vi "Interfaz grafica - corriente.vi"() -> ()   [LabVIEW 2024]
uses:
  160620 Optotune Lens Driver 4 Labview package/Hello Optotune Lens (30.06.2015)/Calibration.ctl
  <vilib>/DAQmx/read.llb/DAQmx Read (Analog 1D Wfm NChan NSamp).vi
  <vilib>/Analysis/2dsp.llb/Decimate (single shot, DBL).vi
  <vilib>/Utility/file.llb/Read Delimited Spreadsheet (string).vi
  <vilib>/Analysis/2dsp.llb/Decimate (continuous, DBL).vi
  <vilib>/Instr/_visa.llb/VISA Configure Serial Port (Instr).vi
  <vilib>/Utility/file.llb/Write Delimited Spreadsheet (string).vi
  <vilib>/DAQmx/create/channels.llb/DAQmx Create Channel (AI-Voltage-Basic).vi
  <vilib>/DAQmx/configure/timing.llb/DAQmx Timing (Sample Clock).vi
  <vilib>/DAQmx/miscellaneous.llb/DAQmx Fill In Error Info.vi
  <vilib>/Waveform/WDTOps.llb/WDT Index Channel DBL.vi
  <vilib>/Waveform/WDTOps.llb/WDT Get Waveform Time Array DBL.vi
  <vilib>/Analysis/NI_AALPro.lvlib
panel:
  out "Array 4":string[](array[string])
  out "Array 3":string[](array[string])
  out "Array 2":string[](array[string])
  out "Array":string[](array[string])
  out "Nombre 2":string
  in  "Restablecer Iniciales":bool
  in  "Incremento":dbl=0.1 format="%#_13g"
  out "Potencia derecho":dbl
  out "error out 4":errorcluster
  out "error out 3":errorcluster
  out "error out 2":errorcluster
  in  "Tab Control 3":enum32{"WL", "Video"}(tab)
  out "Waveform length":dbl[][](graph)
  in  "Minimo escala Y":dbl format="%#_13g"
  in  "Maximo escala Y":dbl format="%#_13g"
  in  "Escala autom. Y":u8=1
  in  "Escala autom. X":u8=1
  in  "Maximo escala X":dbl
  in  "Minimo escala X":dbl
  out "Image Out":T1(plugin-control)
  in  "Frame Rate":u32=30
  in  "Modo de video":u16(ring)=21 items=["160x90 I420 30 fps", "160x90 MJPG 30 fps", "160x90 RGB24 30 fps", "160x120 I420 30 fps", "160x120 MJPG 30 fps", "160x120 RGB24 30 fps", "176x144 I420 30 fps", "176x144 MJPG 30 fps", "176x144 RGB24 30 fps", "320x180 I420 30 fps", "320x180 MJPG 30 fps", "320x180 RGB24 30 fps", "320x240  I420 30 fps", "320x240 MJPG 30 fps", "320x240 RGB24 30 fps", "352x288 I420 30 fps", "352x288 MJPG 30 fps", "352x288 RGB24 30 fps", "432x240 I420 30 fps", "432x240 MJPG 30 fps", "432x240 RGB24 30 fps", "640x360 I420 30 fps", "640x360 MJPG 30 fps", "640x360 RGB24 30 fps", "640x480 I420 30 fps", "640x480 MJPG 30 fps", "640x480 RGB24 30 fps", "800x448 I420 30 fps", "800x448 MJPG 30 fps", "800x448 RGB24 30 fps", "800x600 I420 30 fps", "800x600 MJPG 30 fps", "800x600 RGB24 30 fps", "864x480 I420 30 fps", "864x480 MJPG 30 fps", "864x480 RGB24 30 fps", "960x720 I420 30 fps", "960x720 MJPG 30 fps", "960x720 RGB24 30 fps", "1024x576 I420 30 fps", "1024x576 MJPG 30 fps", "1024x576 RGB24 30 fps", "1280x720 I420 30 fps", "1280x720 MJPG 30 fps", "1280x720 RGB24 30 fps", "1600x896 I420 30 fps", "1600x896 MJPG 30 fps", "1600x896 RGB24 30 fps", "1920x1080 I420 5 fps", "1920x1080 MJPG 30 fps", "1920x1080 RGB24 5 fps", "2304x1296 I420 2 fps", "2304x1296 RGB24 2 fps", "2304x1536 I420 2 fps", "2304x1536 RGB24 2 fps"]
  in  "Carpeta archivo":string="C:\\Users\\TGM1603\\Documents\\LabVIEW Data\\Experimentos electrodos\\VideosExperimentos"
  in  "Calidad":u32=1000
  out "VISA resource name out":string
  in  "Tab Control 2":T2(tab)
  in  "factor decimacion":i32=20
  in  "Ganancia":u16(ring) items=["0.2"=51455, "1"=33023, "10"=49407, "20"=41215, "30"=57599, "40"=37119, "60"=53503, "80"=45311, "120"=61695, "157"=35071, ""=0]
  in  "Potencia inicial lente derecho":dbl(slide) scale=-3.0..3.0
  in  "Potencia inicial lente izquierdo":dbl(slide) scale=-3.0..3.0
  in  "VISA resource name":string="COM11"
  in  "VISA resource name 2":string="COM10"
  out "DPT INICIALES D":dbl
  out "DPT INICIALES I":dbl
  out "Potencia izquierdo":dbl
  in  "error in (no error) 5":errorcluster
  in  "error in (no error) 4":errorcluster
  in  "error in (no error) 3":errorcluster
  in  "error in (no error) 2":errorcluster
  in  "Calibration 4":T3={"Max Current A"=293.0, "Max Current B"=293.0, "UCL A"=300.0, "UCL B"=300.0, "LCL A"=0.0, "LCL B"=0.0} {"Max Current A" format="%#_g mA"; "Max Current B" format="%#_g mA"; "UCL A" format="%#_g mA"; "LCL A" format="%#_g mA"; "UCL B" format="%#_g mA"; "LCL B" format="%#_g mA"}
  out "ID 2":u16
  out "VISA resource name out 2":string
  out "Calibration 3":T3 {"Max Current A" format="%#_g mA"; "Max Current B" format="%#_g mA"; "UCL A" format="%#_g mA"; "LCL A" format="%#_g mA"; "UCL B" format="%#_g mA"; "LCL B" format="%#_g mA"}
  out "OK 2":bool
  out "Data 2":string
  out "Command to Port 2":string
  in  "Cola tipo 2":dbl[](array[numeric])
  out "Distancia":u32
  in  "Tamaño ventana WL":i32=60
  in  "Limite inferior WL":dbl=25.0 format="%#_13g"
  in  "Limite superior WL":dbl=50.0
  out "number":u32
  in  "Calibration":T3={"Max Current A"=293.0, "Max Current B"=293.0, "UCL A"=300.0, "UCL B"=300.0, "LCL A"=0.0, "LCL B"=0.0} {"Max Current A" format="%#_g mA"; "Max Current B" format="%#_g mA"; "UCL A" format="%#_g mA"; "LCL A" format="%#_g mA"; "UCL B" format="%#_g mA"; "LCL B" format="%#_g mA"}
  out "ID":u16
  out "Calibration 2":T3 {"Max Current A" format="%#_g mA"; "Max Current B" format="%#_g mA"; "UCL A" format="%#_g mA"; "LCL A" format="%#_g mA"; "UCL B" format="%#_g mA"; "LCL B" format="%#_g mA"}
  out "OK":bool
  out "Data":string
  out "Command to Port":string
  in  "DPT dif.":dbl
  out "error out":errorcluster
  in  "error in (no error)":errorcluster
  in  "WL":dbl
  in  "Cola tipo":dbl[](array[numeric])
  out "T button?":bool
  in  "Elegir menu Exp":bool
  in  "Elegir menu":bool
  out "path":path
  in  "Iniciar experimento":bool
  in  "Parar adquisicion":bool
  out "Enfermedad visual":string
  out "Edad":string
  out "Nombre":string
  out "Cedula":string
  in  "Carpeta":path=path "C:/Users/TGM1603/Documents/LabVIEW Data/Experimentos electrodos"
  in  "?":bool
  in  "Menu Principal":u16(ring) items=["Visualizacion general ", "Llevar a cabo un experimento", "Ajustar potencia inicial lentes"]
  in  "Menu experimentos":u16(ring) items=["Experimento 1", "Experimento 2", "Experimento 3", "Experimento 4"]
  in  "Tab Control":enum32{"Señal EMG", "Potencia y distancia"}(tab)
  out "Senal EMG":waveform(dbl)[](graph)
  in  "Escala Y min":dbl
  in  "Escala Y max":dbl
  in  "Auto scale Y":u8=1
  in  "Escala X max":dbl
  in  "Escala X min":dbl
  out "Potencia optica y distancia":dbl[][](graph)
  in  "Auto scale X":u8=1
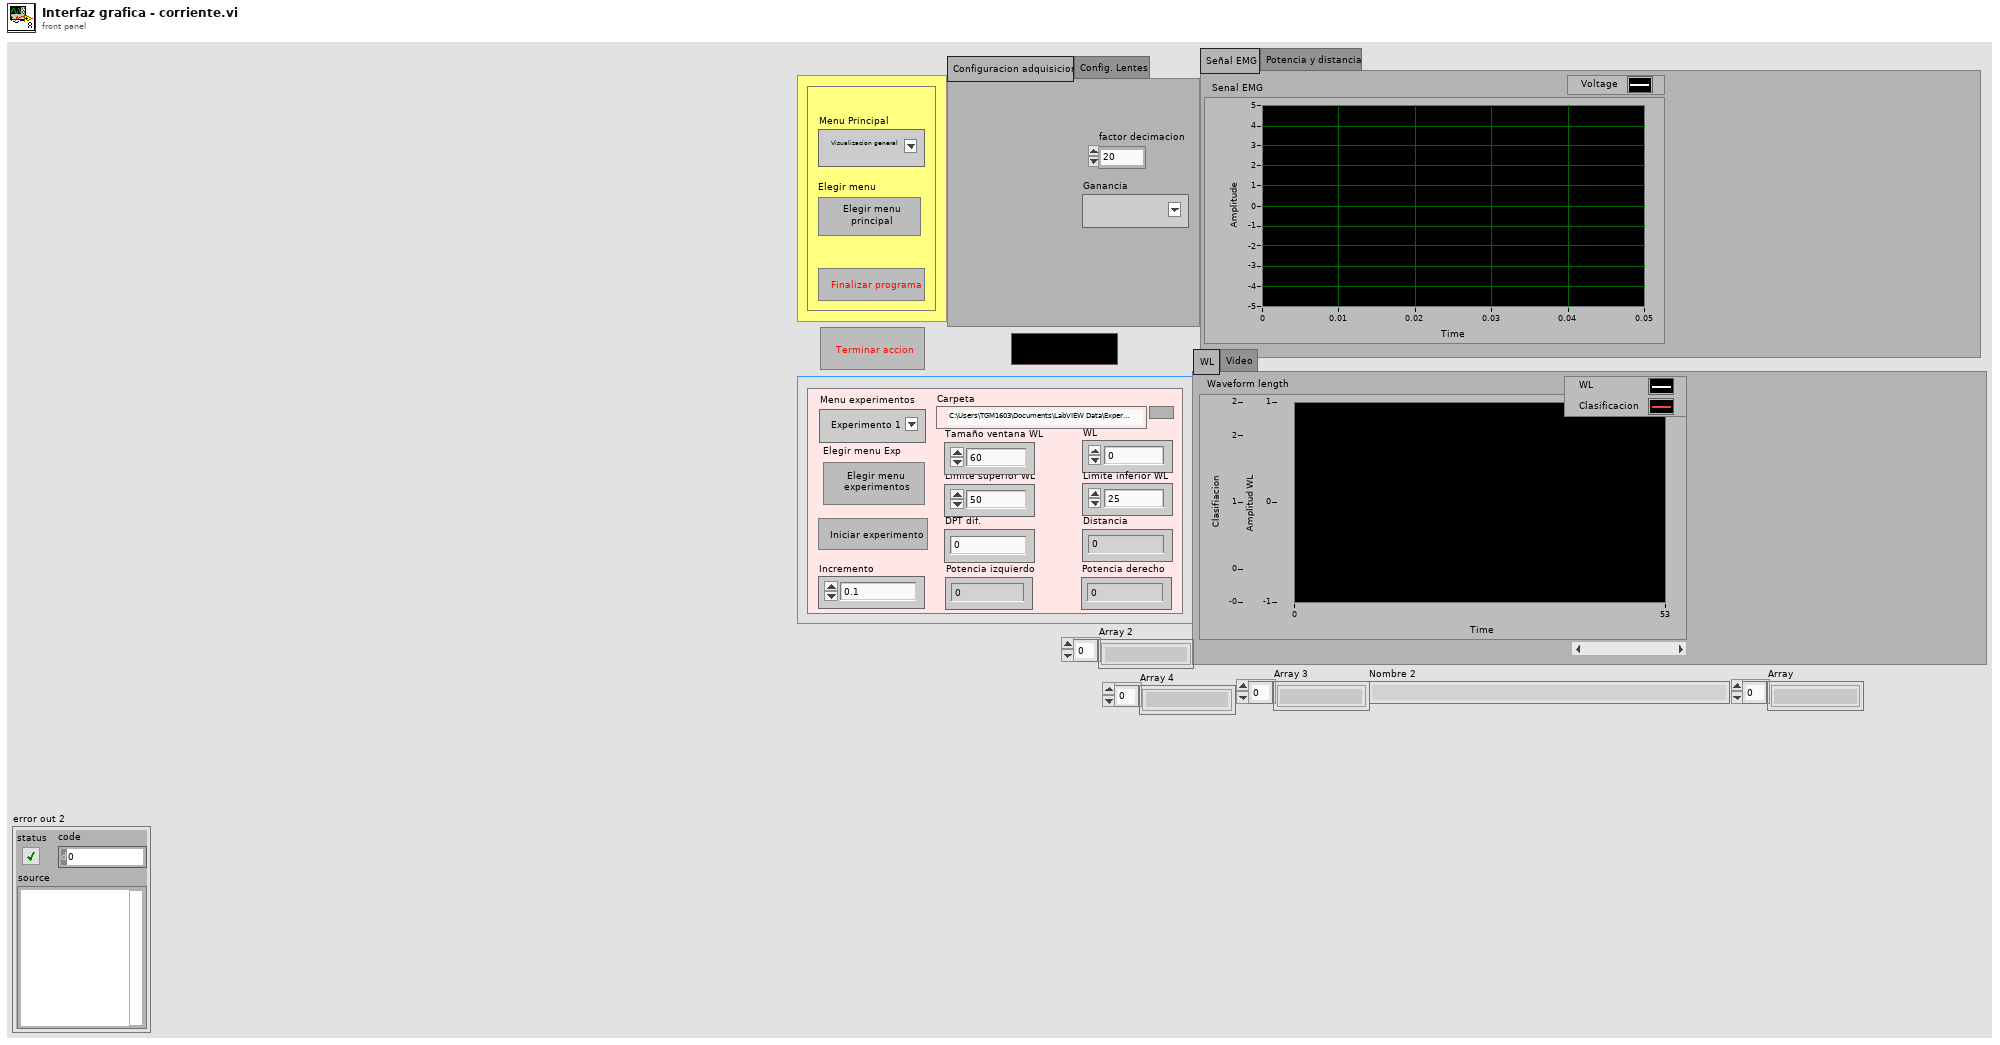
[diagram p1: front panel]
types:
  T1 = typedef "IMAQ Image.ctl" = refnum<image>
  T2 = enum32{"Configuracion adquisicion", "Config. Lentes"}
  T3 = typedef "Calibration.ctl" = cluster{"Max Current A":dbl, "Max Current B":dbl, "UCL A":dbl, "UCL B":dbl, "LCL A":dbl, "LCL B":dbl}
  T4 = enum16{"Left Button", "Center Button", "Right Button", "Window Close"}
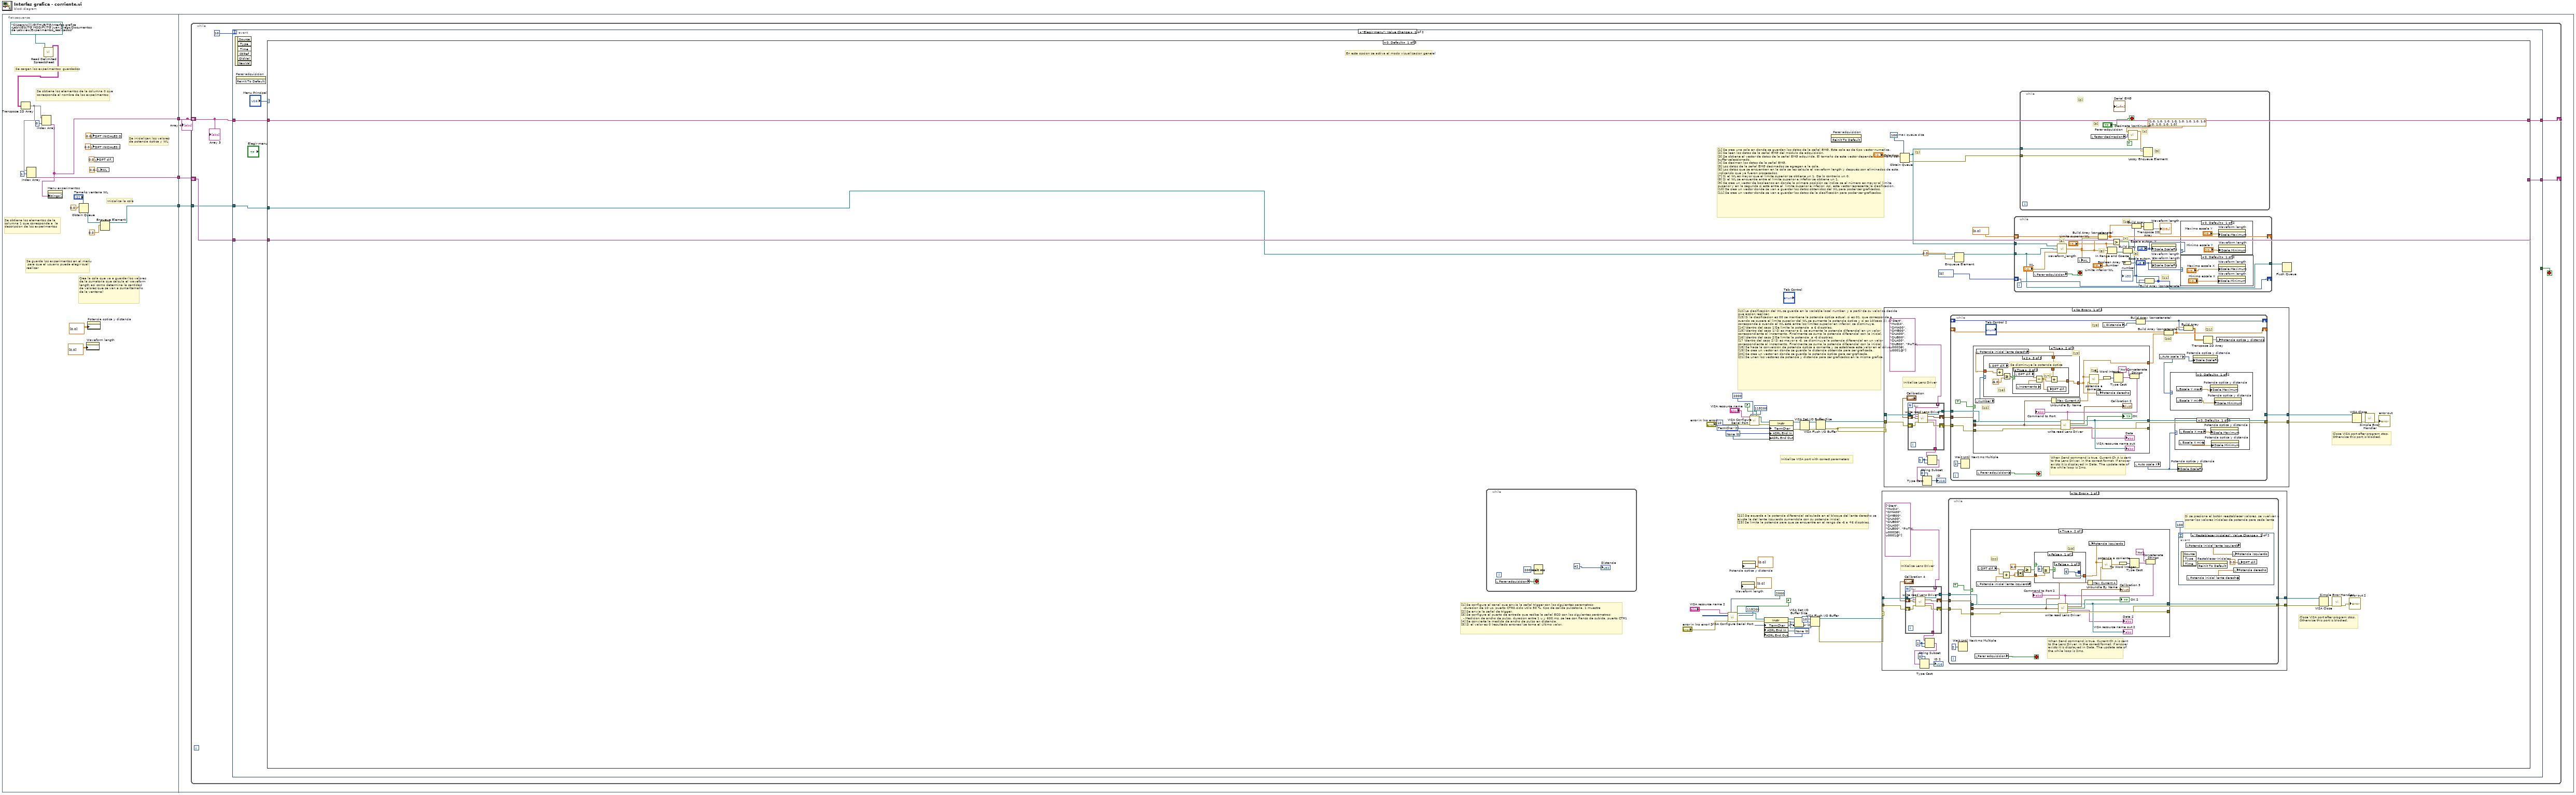
[diagram p0: block diagram]
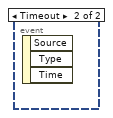
[diagram p2: hidden frame]
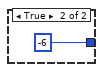
[diagram p4: hidden frame]
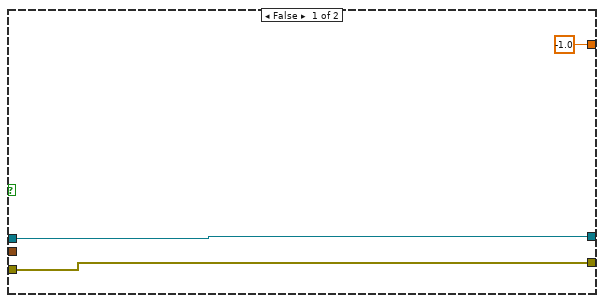
[diagram p9: hidden frame]
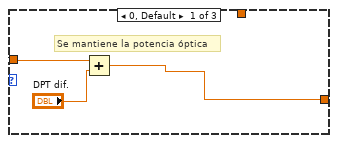
[diagram p10: hidden frame]
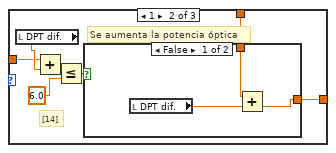
[diagram p11: hidden frame]
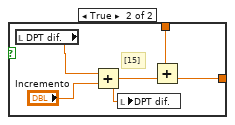
[diagram p12: hidden frame]
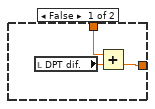
[diagram p13: hidden frame]
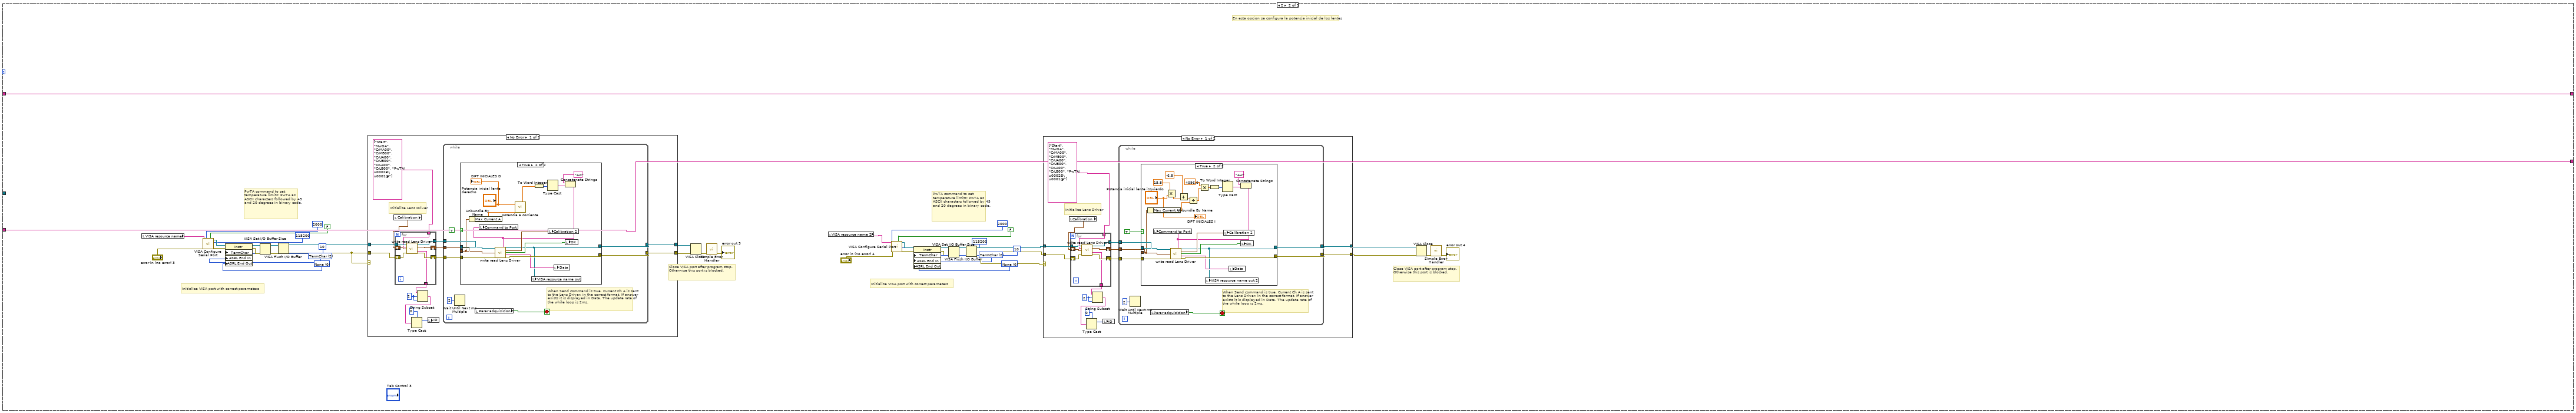
[diagram p17: hidden frame]
diagram:
  n1 = flat-sequence {
    tunnel: [w18] -> w3
    tunnel: [w15] -> w2
    tunnel: [w10] -> w1
    tunnel: w3 -> [w22]
    tunnel: w2 -> [w24]
    tunnel: w1 -> [w23]
    frame #0 {
      # "Se inicializan los valores\nde potencia óptica y WL"
      # "Inicializa la cola"
      # "Crea la cola que va a guardar los valores de la sumatoria que calcula el waveform length así como determina la cantidad de valores que se van a sumar(tamaño de la ventana)"
      # "Se obtiene los elementos de la columna 1 que corresponde a  la descripcion de los experimentos"
      # "Se obtiene los elementos de la columna 0 que corresponde al nombre de los experimentos"
      # "Se guarda los experimentos en el menu\n para que el usuario pueda elegir cual \nrealizar"
      # "Se cargan los experimentos  guardados"
      n2 = call-poly <vilib>:"Read Delimited Spreadsheet.vi"("file path (dialog if empty)"=path "C:/Users/willi/GITHUB/TG/Interfaz grafica -LabVIEW/TG MODIFY/TG Juan Diego/Documentos de Labview/Experimentos_realizados") -> ("all rows"=w19:string[][])  [unwired: 9 in, 5 out]
      n3 = Transpose 2D Array(2D array=w19) -> (transposed array=w16:string[][])
      n4 = Index Array(array=w16, index (row)=1) -> (element=w15:string[])  [unwired: 1 in]
      n5 = Index Array(array=w16, index (row)=0) -> (element=w18:string[])  [unwired: 1 in]
      n6 = property on="Menu experimentos" class="Ring (strict)"("Strings []"=w18) -> ()  [unwired: 2 in, 2 out]
      n7 = Obtain Queue(max queue size (-1, unlimited)="Tamaño ventana WL", element data type=0.0) -> (queue out=w13:refnum<queue>)  [unwired: 3 in, 2 out]
      n8 = property on="Waveform length" class="WFChart (strict)"("History Data"=dbl[][] [[0.0]]) -> ()  [unwired: 2 in, 2 out]
      n9 = property on="Potencia optica y distancia" class="WFChart (strict)"("History Data"=dbl[][] [[0.0]]) -> ()  [unwired: 2 in, 2 out]
      n10 = local write "DPT INICIALES D"(0.0 ("DPT INIT.1")) -> ()
      n11 = local write "DPT INICIALES I"(0.0 ("DPT INIT.2")) -> ()
      n12 = local write "DPT dif."(0.0 ("WL")) -> ()
      n13 = local write "WL"(0.0 ("WL")) -> ()
      n14 = Enqueue Element(queue=w13, element=0.0) -> (queue out=w10:refnum<queue>)  [unwired: 2 in, 2 out]
    }
    frame #1 {
      n15 = while {
        shift-right: [w30] -> _
        shift-left: w22 -> [w31]
        shift-right: [w28] -> _
        shift-left: w24 -> [w29]
        tunnel: w23 -> [w27]
        stop <- w26 stop-if-true
        n16 = event shown="[0] \"Elegir menu\": Value Change" {
          selector: _ -> [_ _]
          dyn-events: _ -> [_ _]
          timeout: 10 -> [_ _]
          tunnel: w31 -> [w37 w982]
          tunnel: [w36 w982] -> w30
          tunnel: w29 -> [w35 w981]
          tunnel: [w34 w981] -> w28
          tunnel: w27 -> [w32 _]
          tunnel: [_ "?"] -> w26
          event "Elegir menu": Value Change {
            n17 = event-data() -> ()  [unwired: 1 in, 6 out]
            n18 = invoke on="Parar adquisicion" class="Bool (strict)" method="Reinit To Default"() -> ()  [unwired: 3 in, 3 out]
            n19 = case shown="0, Default" "Menu Principal" {
              tunnel: w37 -> [w91 w331 w451]
              tunnel: [w91 w331 w450] -> w36
              tunnel: w35 -> [w90 w330 w448]
              tunnel: [w90 w330 w447] -> w34
              tunnel: w32 -> [w85 _ w438]
              frame 0, Default {
                w53 = u16 0 items=["None", "Last Bit", "TermChar", "Break"] ("Serial Settings:End Mode for Writes")
                w52 = u16 2 items=["None", "Last Bit", "TermChar"] ("Serial Settings:End Mode for Reads")
                w75 = u16 0 items=["None", "Last Bit", "TermChar", "Break"] ("Serial Settings:End Mode for Writes")
                w76 = u16 2 items=["None", "Last Bit", "TermChar"] ("Serial Settings:End Mode for Reads")
                w89 = 100  # max queue size
                # "[22] De acuerda a la potencia diferencial calculada en el bloque del lente derecho se ajusta la del lente izquierdo sumandola con su potencia inicial.\n[23] Se limita la potencia para que se encuentre en el rango de -6 a +6 dioptrías."
                # "[12] La clasificación del WL se guarda en la variable local number, y a partir de su valor se decide que accion realizar.\n[13] Si la clasificacion es 00 se mantiene la potencia óptica actual, si es 01, que corresponde a cuando se supera el limite superior del WL,se aumenta la potencia óptica y si es 10(caso 2), que corresponde a cuando el WL está entre los limites superior en inferior, se disminuye. \n[14] (dentro del caso 1)Se limita la potencia  a 6 dioptrías. \n[15] (dentro del caso 1) Si es menor a 6, se aumenta la potencia diferencial en un valor correspondiente al incremento. Finalmente se suma la potencia diferencial con la inicial.\n[16] (dentro del caso 2)Se limita la potencia  a -6 dioptrías.\n[17 (dentro del caso 2) Si es mayor a -6, se disminuye la potencia diferencial en un valor correspondiente al incremento. Finalmente se suma la potencia diferencial con la inicial.\n[18] Se hace la conversión de potencia óptica a corriente y se establece este valor en el driver.\n[19] Se crea un vector en donde se guarda la distancia obtenida para ser graficada.\n[20] Se crea un vector en donde se guarda la potencia óptica para ser graficada.\n[21] Se unen los vectores de potencia y distancia para ser graficados en la misma grafica."
                # "[1] Se crea una cola en donde se guardan los datos de la señal EMG. Esta cola es de tipo vector numerica.\n[2] Se leen los datos de la señal EMG del módulo de adquisición. \n[3] Se obtiene el vector de datos de la señal EMG adquirida. El tamaño de este vector depende del tamaño del buffer seleccionado.\n[4] Se deciman los datos de la señal EMG.\n[5] Los datos de la señal EMG decimados se agregan a la cola.\n[6] Los datos que se encuentran en la cola se les calcula el waveform length y después son eliminados de esta, indicando que ya fueron procesados. \n[7] Si el WL es mayor que el limite superior se obtiene un 1. De lo contrario un 0.\n[8] Si el WL se encuentra entre el límite superior e infefior se obtiene un 1.\n[9] Se crea un vector de booleanos en donde la primera posición se indica se el número es mayor al límite superior y en la segunda si está entre el  limite superior e inferior. Así, este vector representa la clasificación.\n[10] Se crea un vector donde se van a guardar los datos obtenidos del WL para poder ser graficados.\n[11] Se crea un vector donde se van a guardar los datos de la clasificación para poder ser graficados."
                # "[1]"
                # "En esta opcion se activa el modo visualizacion general"
                # "Close VISA port after program stop. Otherwise this port is blocked."
                # "[1] Se configura el canal que envía la señal trigger con los siguientes parametros:\n  -duracion de 10 us, puerto CTR0,ciclo utilo 50 %, tipo de salida pulsatoria, 1 muestra \n[2] Se envía la señal de trigger.\n[3] Se configura el puerto de entrada que recibe la señal ECO con los siguientes parámetros:\n  - Medicion de ancho de pulso, duracion entre 1 u y 600 ms, se lee con flanco de subida, puerto CTR1\n[4] Se convierte la medida de ancho de pulso en distancia.\n[5] Si el valor es 0 (resultado erroneo) se toma el último valor."
                # "Close VISA port after program stop. Otherwise this port is blocked."
                # "Initialize VISA port with correct parameters"
                n20 = while {
                  stop <- w159 stop-if-true
                  n21 = local read "Parar adquisicion"() -> (w159:bool)
                  n22 = Wait (ms)(milliseconds to wait=u32 200) -> ()  [unwired: 1 out]
                  "Distancia" <- 42
                }
                n23 = call-poly "VISA Configure Serial Port"("VISA resource name"="VISA resource name 2", "timeout (10sec)"=u32 2000, "Enable Termination\nChar (T)"=FALSE ("Enable Termination\nChar (T)"), "baud rate (9600)"=u32 115200, "error in (no error)"="error in (no error) 2") -> ("VISA resource name out"=w48:refnum<visa-resource-name>, "error out"=w50:errorcluster)  [unwired: 9 in]
                n24 = property on="Waveform length" class="WFChart (strict)"("History Data"=dbl[][] [[0.0]]) -> ()  [unwired: 2 in, 2 out]
                n25 = property on="Potencia optica y distancia" class="WFChart (strict)"("History Data"=dbl[][] [[0.0]]) -> ()  [unwired: 2 in, 2 out]
                n26 = call-poly "VISA Configure Serial Port"("VISA resource name"="VISA resource name", "timeout (10sec)"=u32 2000, "Enable Termination\nChar (T)"=FALSE ("Enable Termination\nChar (T)"), "baud rate (9600)"=u32 115200, "error in (no error)"="error in (no error)") -> ("VISA resource name out"=w80:refnum<visa-resource-name>, "error out"=w78:errorcluster)  [unwired: 9 in]
                n27 = property class="Instr"(reference=w48, error in=w50, "TermChar"=u8 10 ("Message Based Settings:Termination Character"), "ASRL End In"=w52, "ASRL End Out"=w53) -> (reference out=w49:refnum<visa-resource-name>, error out=w51:errorcluster)
                n28 = property class="Instr"(reference=w80, error in=w78, "TermChar"=u8 10 ("Message Based Settings:Termination Character"), "ASRL End In"=w76, "ASRL End Out"=w75) -> (reference out=w79:refnum<visa-resource-name>, error out=w77:errorcluster)
                n29 = VISA Set I/O Buffer Size(VISA resource name=w49, error in (no error)=w51) -> (VISA resource name out=w56:refnum<visa-resource-name>, error out=w57:errorcluster)  [unwired: 2 in]
                n30 = VISA Set I/O Buffer Size(VISA resource name=w79, error in (no error)=w77) -> (VISA resource name out=w72:refnum<visa-resource-name>, error out=w71:errorcluster)  [unwired: 2 in]
                n31 = VISA Flush I/O Buffer(VISA resource name=w56, error in (no error)=w57) -> (VISA resource name out=w42:refnum<visa-resource-name>, error out=w43:errorcluster)  [unwired: 1 in]
                n32 = VISA Flush I/O Buffer(VISA resource name=w72, error in (no error)=w71) -> (VISA resource name out=w70:refnum<visa-resource-name>, error out=w65:errorcluster)  [unwired: 1 in]
                n33 = invoke on="Parar adquisicion" class="Bool (strict)" method="Reinit To Default"() -> ()  [unwired: 3 in, 3 out]
                n34 = case shown="No Error" w43 {
                  tunnel: w43 -> [w105 w156]
                  tunnel: w42 -> [w104 w157]
                  tunnel: [w103 w156] -> w38
                  tunnel: [w102 w157] -> w39
                  frame No Error {
                    w100 = 2 ("length (rest)")
                    # "Initialize Lens Driver"
                    n35 = for {
                      tunnel: w104 -> [w154]
                      tunnel: [w151] -> w94
                      tunnel: string[] ["Start", "MwDA", "CrMA00", "CrMB00", "CrUA00", "CrUB00", "CrLA00", "CrLB00", "PwTA\u0002Ð\u0001@"] -> [w149] mode=indexing
                      tunnel: [w148] -> w93
                      shift-right: [w152] -> w95
                      shift-left: "Calibration 4" -> [w153]
                      shift-right: [w150] -> w96
                      shift-left: w105 -> [w155]
                      n36 = call "write read Lens Driver.vi"("VISA resource name"=w154, "command"=w149, "Calibration"=w153, "error in (no error)"=w155) -> ("VISA resource name out"=w151:refnum<visa-resource-name>, "Calibration 2"=w152:T3, "Data"=w148:string, "error out"=w150:errorcluster)  [unwired: 4 in, 4 out]
                    }
                    n37 = String Subset(string=w93, offset (0)=w100, length (rest)=w100) -> (substring=w98:string)
                    n38 = Type Cast(type=u16 0 ("length (rest)"), x=w98) -> (*(type *) &x=→"ID 2":u16)
                    n39 = while {
                      tunnel: [w108] -> w103
                      tunnel: [w109] -> w102
                      tunnel: w96 -> [w114]
                      tunnel: w95 -> [w113]
                      tunnel: w94 -> [w112]
                      stop <- w107 stop-if-true
                      # "Si se presiona el botón reestablecer valores, se vuelven a poner los valores iniciales de potencia para cada lente"
                      # "When Send command is true, Current Ch A is sent to the Lens Driver, in the correct format. If answer exists it is displayed in Data. The update rate of the while loop is 2ms."
                      n40 = Wait Until Next ms Multiple(millisecond multiple=u32 2) -> ()  [unwired: 1 out]
                      n41 = case shown="True" TRUE ("Send command") {
                        tunnel: [w119 w140] -> w108
                        tunnel: w114 -> [w119 w139]
                        tunnel: w113 -> [_ w121]
                        tunnel: w112 -> [w118 w138]
                        tunnel: [w118 w135] -> w109
                        frame False {
                        }
                        frame True {
                          # "[23]"
                          # "[22]"
                          n42 = local read "Potencia inicial lente izquierdo"() -> (w129:dbl)
                          n43 = local read "DPT dif."() -> (w130:dbl)
                          n44 = Add(x=w130, y=w129) -> (x+y=w125:dbl)
                          n45 = Absolute Value(x=w125) -> (abs(x)=w127:dbl)
                          n46 = Greater Or Equal?(x=6.0, y=w127) -> (x >= y?=w128:bool)
                          n47 = case shown="False" w128 {
                            tunnel: w125 -> [w143 w147]
                            tunnel: [w141 w147] -> w123
                            frame False {
                              n48 = Greater Or Equal?(x=u16 0, y=w143) -> (x >= y?=w144:bool)
                              n49 = case shown="False" w144 {
                                tunnel: [i16 6 ("x") i16 -6 ("x")] -> w141
                                frame False {
                                }
                                frame True {
                                }
                              }
                            }
                            frame True {
                            }
                          }
                          n50 = Unbundle By Name(w121) -> ("Max Current A"=w122:dbl)
                          n51 = local write "Potencia izquierdo"(w123) -> ()
                          n52 = call "potencia a corriente.vi"("Max current A"=w122, "Potencia"=w123) -> ("Corriente"=w124:dbl)
                          n53 = To Word Integer(number=w124) -> (16bit integer=w133:i16)
                          n54 = Type Cast(x=w133) -> (*(type *) &x=w132:string)  [unwired: 1 in]
                          n55 = Concatenate Strings("Aw", w132) -> (w131:string)
                          "Command to Port 2" <- w131
                          n56 = call "write read Lens Driver.vi"("VISA resource name"=w138, "command"=w131, "Calibration"=w121, "error in (no error)"=w139) -> ("VISA resource name out"=w135:refnum<visa-resource-name>, "Calibration 2"=→"Calibration 3":T3, "OK"=→"OK 2":bool, "Data"=→"Data 2":string, "error out"=w140:errorcluster)  [unwired: 4 in, 3 out]
                          "VISA resource name out 2" <- w135
                        }
                      }
                      n57 = local read "Parar adquisicion"() -> (w107:bool)
                      n58 = event shown="[0] \"Restablecer Iniciales\": Value Change" {
                        selector: _ -> [_ _]
                        dyn-events: _ -> [_ _]
                        timeout: 100 -> [_ _]
                        event "Restablecer Iniciales": Value Change {
                          n59 = event-data() -> ()  [unwired: 1 in, 3 out]
                          n60 = local read "Potencia inicial lente izquierdo"() -> (w115:dbl)
                          n61 = local read "Potencia inicial lente derecho"() -> (w116:dbl)
                          n62 = invoke on="Restablecer Iniciales" class="Bool" method="Reinit To Default"() -> ()  [unwired: 3 in, 3 out]
                          n63 = local write "Potencia izquierdo"(w115) -> ()
                          n64 = local write "Potencia derecho"(w116) -> ()
                          n65 = local write "DPT dif."(0.0 ("DPT dif.")) -> ()
                        }
                        event Timeout {
                          n66 = event-data() -> ()  [unwired: 1 in, 3 out]
                        }
                      }
                    }
                  }
                  frame Error {
                  }
                }
                n67 = case shown="No Error" w65 {
                  tunnel: w65 -> [w174 w258]
                  tunnel: w70 -> [w173 w259]
                  tunnel: [w172 w258] -> w68
                  tunnel: [w171 w259] -> w66
                  frame No Error {
                    w169 = 2 ("length (rest)")
                    # "Initialize Lens Driver"
                    n68 = for {
                      tunnel: w173 -> [w256]
                      tunnel: [w253] -> w163
                      tunnel: string[] ["Start", "MwDA", "CrMA00", "CrMB00", "CrUA00", "CrUB00", "CrLA00", "CrLB00", "PwTA\u0002Ð\u0001@"] -> [w251] mode=indexing
                      tunnel: [w250] -> w162
                      shift-right: [w254] -> w164
                      shift-left: "Calibration" -> [w255]
                      shift-right: [w252] -> w165
                      shift-left: w174 -> [w257]
                      n69 = call "write read Lens Driver.vi"("VISA resource name"=w256, "command"=w251, "Calibration"=w255, "error in (no error)"=w257) -> ("VISA resource name out"=w253:refnum<visa-resource-name>, "Calibration 2"=w254:T3, "Data"=w250:string, "error out"=w252:errorcluster)  [unwired: 4 in, 4 out]
                    }
                    n70 = String Subset(string=w162, offset (0)=w169, length (rest)=w169) -> (substring=w167:string)
                    n71 = Type Cast(type=u16 0 ("length (rest)"), x=w167) -> (*(type *) &x=→"ID":u16)
                    n72 = while {
                      tunnel: [w186] -> w172
                      tunnel: [w187] -> w171
                      tunnel: w165 -> [w192]
                      tunnel: w164 -> [w191]
                      tunnel: w163 -> [w190]
                      shift-right: [w177] -> _
                      shift-left: _ -> [w181]
                      shift-right: [w178] -> _
                      shift-left: _ -> [w180]
                      stop <- w185 stop-if-true
                      # "[21]"
                      # "[20]"
                      # "[19]"
                      # "When Send command is true, Current Ch A is sent to the Lens Driver, in the correct format. If answer exists it is displayed in Data. The update rate of the while loop is 2ms."
                      n73 = Wait Until Next ms Multiple(millisecond multiple=u32 2) -> ()  [unwired: 1 out]
                      n74 = case shown="True" TRUE ("Send command") {
                        tunnel: [w199 w216] -> w186
                        tunnel: w192 -> [w199 w215]
                        tunnel: w191 -> [_ w202]
                        tunnel: w190 -> [w198 w214]
                        tunnel: [w198 w211] -> w187
                        tunnel: [-1.0 ("DPT") w204] -> w179
                        frame False {
                        }
                        frame True {
                          # "[18]"
                          # "[13]"
                          # "[12]"
                          n75 = local read "number"() -> (w206:u32)
                          n76 = local read "Potencia inicial lente derecho"() -> (w205:dbl)
                          n77 = case shown="2" w206 {
                            tunnel: [w218 w226 w241] -> w204
                            tunnel: w205 -> [w219 w221 w236]
                            tunnel: w205 -> [_ w220 w235]
                            frame 0, Default {
                              # "Se mantiene la potencia óptica"
                              n78 = Add(x=w219, y="DPT dif.") -> (x+y=w218:dbl)
                            }
                            frame 1 {
                              # "[14]"
                              # "Se aumenta la potencia óptica"
                              n79 = local read "DPT dif."() -> (w222:dbl)
                              n80 = Add(x=w221, y=w222) -> (x+y=w223:dbl)
                              n81 = Less Or Equal?(x=w223, y=6.0) -> (x <= y?=w225:bool)
                              n82 = case shown="False" w225 {
                                tunnel: [w228 w231] -> w226
                                tunnel: w220 -> [w227 w230]
                                frame False {
                                n83 = local read "DPT dif."() -> (w229:dbl)
                                n84 = Add(x=w227, y=w229) -> (x+y=w228:dbl)
                                }
                                frame True {
                                # "[15]"
                                n85 = local read "DPT dif."() -> (w232:dbl)
                                n86 = Add(x=w232, y="Incremento") -> (x+y=w233:dbl)
                                n87 = local write "DPT dif."(w233) -> ()
                                n88 = Add(x=w230, y=w233) -> (x+y=w231:dbl)
                                }
                              }
                            }
                            frame 2 {
                              # "[16]"
                              # "Se disminuye la potencia óptica"
                              n89 = local read "DPT dif."() -> (w240:dbl)
                              n90 = Add(x=w240, y=w236) -> (x+y=w237:dbl)
                              n91 = Greater Or Equal?(x=w237, y=-6.0) -> (x >= y?=w238:bool)
                              n92 = case shown="True" w238 {
                                tunnel: [w243 w247] -> w241
                                tunnel: w235 -> [w242 w246]
                                frame False {
                                n93 = local read "DPT dif."() -> (w244:dbl)
                                n94 = Add(x=w242, y=w244) -> (x+y=w243:dbl)
                                }
                                frame True {
                                # "[17]"
                                n95 = local read "DPT dif."() -> (w249:dbl)
                                n96 = local read "Incremento"() -> (w245:dbl)
                                n97 = Subtract(x=w249, y=w245) -> (x-y=w248:dbl)
                                n98 = local write "DPT dif."(w248) -> ()
                                n99 = Add(x=w246, y=w248) -> (x+y=w247:dbl)
                                }
                              }
                            }
                          }
                          n100 = Unbundle By Name(w202) -> ("Max Current A"=w201:dbl)
                          n101 = call "potencia a corriente.vi"("Max current A"=w201, "Potencia"=w204) -> ("Corriente"=w203:dbl)
                          n102 = local write "Potencia derecho"(w204) -> ()
                          n103 = To Word Integer(number=w203) -> (16bit integer=w209:i16)
                          n104 = Type Cast(x=w209) -> (*(type *) &x=w208:string)  [unwired: 1 in]
                          n105 = Concatenate Strings("Aw", w208) -> (w207:string)
                          "Command to Port" <- w207
                          n106 = call "write read Lens Driver.vi"("VISA resource name"=w214, "command"=w207, "Calibration"=w202, "error in (no error)"=w215) -> ("VISA resource name out"=w211:refnum<visa-resource-name>, "Calibration 2"=→"Calibration 2":T3, "OK"=→"OK":bool, "Data"=→"Data":string, "error out"=w216:errorcluster)  [unwired: 4 in, 3 out]
                          "VISA resource name out" <- w211
                        }
                      }
                      n107 = local read "Parar adquisicion"() -> (w185:bool)
                      n108 = local read "Distancia"() -> (w182:u32)
                      n109 = local read "Auto scale X"() -> (w183:u8)
                      n110 = Build Array (concatenate)(w181, w182) -> (w177:u32[])
                      n111 = local read "Auto scale Y"() -> (w184:u8)
                      n112 = Build Array (concatenate)(w180, w179) -> (w178:dbl[])
                      n113 = case shown="0, Default" w184 {
                        frame 0, Default {
                          n114 = local read "Escala Y max"() -> (w196:dbl)
                          n115 = local read "Escala Y min"() -> (w195:dbl)
                          n116 = property on="Potencia optica y distancia" class="WFChart (strict)"("YScale.Maximum"=w196) -> ()  [unwired: 2 in, 2 out]
                          n117 = property on="Potencia optica y distancia" class="WFChart (strict)"("YScale.Minimum"=w195) -> ()  [unwired: 2 in, 2 out]
                        }
                        frame 1 {
                        }
                      }
                      n118 = case shown="0, Default" w183 {
                        frame 0, Default {
                          n119 = local read "Escala X min"() -> (w193:dbl)
                          n120 = local read "Escala X max"() -> (w194:dbl)
                          n121 = property on="Potencia optica y distancia" class="WFChart (strict)"("XScale.Maximum"=w194) -> ()  [unwired: 2 in, 2 out]
                          n122 = property on="Potencia optica y distancia" class="WFChart (strict)"("XScale.Minimum"=w193) -> ()  [unwired: 2 in, 2 out]
                        }
                        frame 1 {
                        }
                      }
                      n123 = property on="Potencia optica y distancia" class="WFChart (strict)"("XScale.ScaleFit"=w183) -> ()  [unwired: 2 in, 2 out]
                      n124 = Build Array(w178, w177) -> (w176:dbl[][])
                      n125 = property on="Potencia optica y distancia" class="WFChart (strict)"("YScale.ScaleFit"=w184) -> ()  [unwired: 2 in, 2 out]
                      n126 = Transpose 2D Array(2D array=w176) -> (transposed array=w175:dbl[][])
                      n127 = local write "Potencia optica y distancia"(w175) -> ()
                    }
                  }
                  frame Error {
                  }
                }
                n128 = Obtain Queue(max queue size (-1, unlimited)=w89, element data type="Cola tipo") -> (queue out=w86:refnum<queue>, error out=w87:errorcluster)  [unwired: 3 in, 1 out]
                n129 = Enqueue Element(queue=w85, element=0.0) -> (queue out=w62:refnum<queue>)  [unwired: 2 in, 2 out]
                n130 = while {
                  tunnel: w62 -> [w261]
                  tunnel: w86 -> [w278]
                  shift-right: [w264] -> _
                  shift-left: dbl[] [0.0] -> [w275]
                  shift-right: [w263] -> _
                  shift-left: u32[] [0] -> [w265]
                  tunnel: [w261] -> w60
                  stop <- w276 stop-if-true
                  # "[11]"
                  # "[10]"
                  # "[9]"
                  # "[8]"
                  # "[7]"
                  # "[6]"
                  n131 = local read "Parar adquisicion"() -> (w276:bool)
                  n132 = call "waveform_length.vi"("WL"="WL", "Cola WL"=w261, "Datos entrada"=w278) -> ("WL 2"=w273:dbl)
                  n133 = local write "WL"(w273) -> ()
                  n134 = Build Array (concatenate)(w275, w273) -> (w264:dbl[])
                  n135 = In Range and Coerce(upper limit="Limite superior WL", x=w273, lower limit="Limite inferior WL") -> (In Range?=w271:bool)  [unwired: 1 out]
                  n136 = Greater?(x=w273, y="Limite superior WL") -> (0:w272:bool)
                  n137 = Build Array(w272, w271) -> (w270:bool[])
                  n138 = Boolean Array To Number(Boolean array=w270) -> (number=w266:u32)
                  "number" <- w266
                  n139 = Build Array (concatenate)(w265, w266) -> (w263:u32[])
                  n140 = Build Array(w264, w263) -> (w262:dbl[][])
                  n141 = Transpose 2D Array(2D array=w262) -> (transposed array=→"Waveform length":dbl[][])
                  n142 = property on="Waveform length" class="WFChart (strict)"("YScale.ScaleFit"="Escala autom. Y") -> ()  [unwired: 2 in, 2 out]
                  n143 = property on="Waveform length" class="WFChart (strict)"("XScale.ScaleFit"="Escala autom. X") -> ()  [unwired: 2 in, 2 out]
                  n144 = case shown="0, Default" "Escala autom. Y" {
                    frame 0, Default {
                      n145 = property on="Waveform length" class="WFChart (strict)"("YScale.Maximum"="Maximo escala Y") -> ()  [unwired: 2 in, 2 out]
                      n146 = property on="Waveform length" class="WFChart (strict)"("YScale.Minimum"="Minimo escala Y") -> ()  [unwired: 2 in, 2 out]
                    }
                    frame 1 {
                    }
                  }
                  n147 = case shown="0, Default" "Escala autom. X" {
                    frame 0, Default {
                      n148 = property on="Waveform length" class="WFChart (strict)"("XScale.Minimum"="Minimo escala X") -> ()  [unwired: 2 in, 2 out]
                      n149 = property on="Waveform length" class="WFChart (strict)"("XScale.Maximum"="Maximo escala X") -> ()  [unwired: 2 in, 2 out]
                    }
                    frame 1 {
                    }
                  }
                }
                n150 = while {
                  tunnel: w86 -> [w287]
                  tunnel: w87 -> [w286]
                  stop <- "Parar adquisicion" stop-if-true
                  # "[5]"
                  # "[4]"
                  # "[3]"
                  # "[2]"
                  n151 = local read "factor decimacion"() -> (w288:i32)
                  n152 = call-poly <vilib>:"Decimate (continuous).vi"("averaging"=TRUE, "decimating factor"=w288, "X"=dbl[] [1.0, 1.0, 1.0, 1.0, 1.0, 1.0, 1.0, 1.0, 1.0, 1.0, 1.0, 1.0] ("Decimated Array")) -> ("Decimated Array"=w285:dbl[])  [unwired: 7 in, 1 out]
                  n153 = Lossy Enqueue Element(queue=w287, element=w285, error in (no error)=w286) -> ()  [unwired: 4 out]
                }
                n154 = Flush Queue(queue=w60) -> ()  [unwired: 1 in, 3 out]
                n155 = VISA Close(VISA resource name=w39, error in (no error)=w38) -> (error out=w40:errorcluster)
                n156 = call <vilib>:"Simple Error Handler.vi"("error in (no error)"=w40) -> ("error out"=→"error out 2":errorcluster)  [unwired: 4 in, 4 out]
                n157 = VISA Close(VISA resource name=w66, error in (no error)=w68) -> (error out=w69:errorcluster)
                n158 = call <vilib>:"Simple Error Handler.vi"("error in (no error)"=w69) -> ("error out"=→"error out":errorcluster)  [unwired: 4 in, 4 out]
              }
              frame 2 {
                w310 = u16 0 items=["None", "Last Bit", "TermChar", "Break"] ("Serial Settings:End Mode for Writes")
                w309 = u16 2 items=["None", "Last Bit", "TermChar"] ("Serial Settings:End Mode for Reads")
                w323 = u16 0 items=["None", "Last Bit", "TermChar", "Break"] ("Serial Settings:End Mode for Writes")
                w322 = u16 2 items=["None", "Last Bit", "TermChar"] ("Serial Settings:End Mode for Reads")
                # "En esta opcion se configura la potencia inicial de los lentes"
                # "Close VISA port after program stop. Otherwise this port is blocked."
                # "Close VISA port after program stop. Otherwise this port is blocked."
                # "PwTA command to set temperature limits: PwTA as ASCII characters followed by 45 and 20 degrees in binary code."
                # "Initialize VISA port with correct parameters"
                # "PwTA command to set temperature limits: PwTA as ASCII characters followed by 45 and 20 degrees in binary code."
                # "Initialize VISA port with correct parameters"
                n159 = local read "VISA resource name"() -> (w300:string)
                n160 = call-poly "VISA Configure Serial Port"("VISA resource name"=w300, "timeout (10sec)"=u32 2000, "Enable Termination\nChar (T)"=FALSE ("Enable Termination\nChar (T)"), "baud rate (9600)"=u32 115200, "error in (no error)"="error in (no error) 3") -> ("VISA resource name out"=w305:refnum<visa-resource-name>, "error out"=w307:errorcluster)  [unwired: 9 in]
                n161 = property class="Instr"(reference=w305, error in=w307, "TermChar"=u8 10 ("Message Based Settings:Termination Character"), "ASRL End In"=w309, "ASRL End Out"=w310) -> (reference out=w306:refnum<visa-resource-name>, error out=w308:errorcluster)
                n162 = VISA Set I/O Buffer Size(VISA resource name=w306, error in (no error)=w308) -> (VISA resource name out=w312:refnum<visa-resource-name>, error out=w313:errorcluster)  [unwired: 2 in]
                n163 = VISA Flush I/O Buffer(VISA resource name=w312, error in (no error)=w313) -> (VISA resource name out=w299:refnum<visa-resource-name>, error out=w298:errorcluster)  [unwired: 1 in]
                n164 = case shown="No Error" w298 {
                  tunnel: w298 -> [w345 w379]
                  tunnel: w299 -> [w344 w380]
                  tunnel: [w343 w379] -> w294
                  tunnel: [w342 w380] -> w295
                  frame No Error {
                    w341 = 2 ("length (rest)")
                    # "Initialize Lens Driver"
                    n165 = local read "Calibration"() -> (w333:T3)
                    n166 = for {
                      tunnel: w344 -> [w377]
                      tunnel: [w374] -> w336
                      tunnel: string[] ["Start", "MwDA", "CrMA00", "CrMB00", "CrUA00", "CrUB00", "CrLA00", "CrLB00", "PwTA\u0002Ð\u0001@"] -> [w372] mode=indexing
                      tunnel: [w371] -> w335
                      shift-right: [w375] -> w337
                      shift-left: w333 -> [w376]
                      shift-right: [w373] -> w338
                      shift-left: w345 -> [w378]
                      n167 = call "write read Lens Driver.vi"("VISA resource name"=w377, "command"=w372, "Calibration"=w376, "error in (no error)"=w378) -> ("VISA resource name out"=w374:refnum<visa-resource-name>, "Calibration 2"=w375:T3, "Data"=w371:string, "error out"=w373:errorcluster)  [unwired: 4 in, 4 out]
                    }
                    n168 = String Subset(string=w335, offset (0)=w341, length (rest)=w341) -> (substring=w339:string)
                    n169 = Type Cast(type=u16 0 ("length (rest)"), x=w339) -> (*(type *) &x=w334:u16)
                    n170 = local write "ID"(w334) -> ()
                    n171 = while {
                      tunnel: [w347] -> w343
                      tunnel: [w348] -> w342
                      tunnel: w338 -> [w353]
                      tunnel: w337 -> [w352]
                      tunnel: w336 -> [w351]
                      stop <- w346 stop-if-true
                      # "When Send command is true, Current Ch A is sent to the Lens Driver, in the correct format. If answer exists it is displayed in Data. The update rate of the while loop is 2ms."
                      n172 = Wait Until Next ms Multiple(millisecond multiple=u32 2) -> ()  [unwired: 1 out]
                      n173 = case shown="True" TRUE ("Send command") {
                        tunnel: [w355 w370] -> w347
                        tunnel: w353 -> [w355 w369]
                        tunnel: w352 -> [_ w360]
                        tunnel: w351 -> [w354 w368]
                        tunnel: [w354 w361] -> w348
                        frame False {
                        }
                        frame True {
                          n174 = Unbundle By Name(w360) -> ("Max Current A"=w359:dbl)
                          n175 = call "potencia a corriente.vi"("Max current A"=w359, "Potencia"="Potencia inicial lente derecho") -> ("Corriente"=w357:dbl)
                          n176 = To Word Integer(number=w357) -> (16bit integer=w367:i16)
                          n177 = Type Cast(x=w367) -> (*(type *) &x=w366:string)  [unwired: 1 in]
                          n178 = Concatenate Strings("Aw", w366) -> (w363:string)
                          n179 = local write "Command to Port"(w363) -> ()
                          n180 = call "write read Lens Driver.vi"("VISA resource name"=w368, "command"=w363, "Calibration"=w360, "error in (no error)"=w369) -> ("VISA resource name out"=w361:refnum<visa-resource-name>, "Calibration 2"=w365:T3, "OK"=w364:bool, "Data"=w362:string, "error out"=w370:errorcluster)  [unwired: 4 in, 3 out]
                          n181 = local write "VISA resource name out"(w361) -> ()
                          n182 = local write "Calibration 2"(w365) -> ()
                          n183 = local write "Data"(w362) -> ()
                          n184 = local write "OK"(w364) -> ()
                          "DPT INICIALES D" <- "Potencia inicial lente derecho"
                        }
                      }
                      n185 = local read "Parar adquisicion"() -> (w346:bool)
                    }
                  }
                  frame Error {
                  }
                }
                n186 = VISA Close(VISA resource name=w295, error in (no error)=w294) -> (error out=w297:errorcluster)
                n187 = call <vilib>:"Simple Error Handler.vi"("error in (no error)"=w297) -> ("error out"=→"error out 3":errorcluster)  [unwired: 4 in, 4 out]
                n188 = local read "VISA resource name 2"() -> (w314:string)
                n189 = call-poly "VISA Configure Serial Port"("VISA resource name"=w314, "timeout (10sec)"=u32 2000, "Enable Termination\nChar (T)"=FALSE ("Enable Termination\nChar (T)"), "baud rate (9600)"=u32 115200, "error in (no error)"="error in (no error) 4") -> ("VISA resource name out"=w318:refnum<visa-resource-name>, "error out"=w320:errorcluster)  [unwired: 9 in]
                n190 = property class="Instr"(reference=w318, error in=w320, "TermChar"=u8 10 ("Message Based Settings:Termination Character"), "ASRL End In"=w322, "ASRL End Out"=w323) -> (reference out=w319:refnum<visa-resource-name>, error out=w321:errorcluster)
                n191 = VISA Set I/O Buffer Size(VISA resource name=w319, error in (no error)=w321) -> (VISA resource name out=w325:refnum<visa-resource-name>, error out=w326:errorcluster)  [unwired: 2 in]
                n192 = VISA Flush I/O Buffer(VISA resource name=w325, error in (no error)=w326) -> (VISA resource name out=w328:refnum<visa-resource-name>, error out=w327:errorcluster)  [unwired: 1 in]
                n193 = case shown="No Error" w327 {
                  tunnel: w327 -> [w394 w434]
                  tunnel: w328 -> [w393 w435]
                  tunnel: [w392 w434] -> w291
                  tunnel: [w391 w435] -> w290
                  frame No Error {
                    w390 = 2 ("length (rest)")
                    # "Initialize Lens Driver"
                    n194 = local read "Calibration"() -> (w382:T3)
                    n195 = for {
                      tunnel: w393 -> [w432]
                      tunnel: [w429] -> w385
                      tunnel: string[] ["Start", "MwDA", "CrMA00", "CrMB00", "CrUA00", "CrUB00", "CrLA00", "CrLB00", "PwTA\u0002Ð\u0001@"] -> [w427] mode=indexing
                      tunnel: [w426] -> w384
                      shift-right: [w430] -> w386
                      shift-left: w382 -> [w431]
                      shift-right: [w428] -> w387
                      shift-left: w394 -> [w433]
                      n196 = call "write read Lens Driver.vi"("VISA resource name"=w432, "command"=w427, "Calibration"=w431, "error in (no error)"=w433) -> ("VISA resource name out"=w429:refnum<visa-resource-name>, "Calibration 2"=w430:T3, "Data"=w426:string, "error out"=w428:errorcluster)  [unwired: 4 in, 4 out]
                    }
                    n197 = String Subset(string=w384, offset (0)=w390, length (rest)=w390) -> (substring=w388:string)
                    n198 = Type Cast(type=u16 0 ("length (rest)"), x=w388) -> (*(type *) &x=w383:u16)
                    n199 = local write "ID"(w383) -> ()
                    n200 = while {
                      tunnel: [w396] -> w392
                      tunnel: [w397] -> w391
                      tunnel: w387 -> [w402]
                      tunnel: w386 -> [w401]
                      tunnel: w385 -> [w400]
                      stop <- w395 stop-if-true
                      # "When Send command is true, Current Ch A is sent to the Lens Driver, in the correct format. If answer exists it is displayed in Data. The update rate of the while loop is 2ms."
                      n201 = Wait Until Next ms Multiple(millisecond multiple=u32 2) -> ()  [unwired: 1 out]
                      n202 = case shown="True" TRUE ("Send command") {
                        tunnel: [w404 w425] -> w396
                        tunnel: w402 -> [w404 w424]
                        tunnel: w401 -> [_ w412]
                        tunnel: w400 -> [w403 w423]
                        tunnel: [w403 w413] -> w397
                        frame False {
                        }
                        frame True {
                          n203 = Unbundle By Name(w412) -> ("Max Current A"=w411:dbl)
                          n204 = Multiply(x=15.8, y="Potencia inicial lente izquierdo") -> (x*y=w409:dbl)
                          n205 = Add(x=-6.8, y=w409) -> (x+y=w407:dbl)
                          n206 = Divide(x=w407, y=w411) -> (x/y=w410:dbl)
                          n207 = Multiply(x=4096.0, y=w410) -> (x*y=w421:dbl)
                          n208 = To Word Integer(number=w421) -> (16bit integer=w420:i16)
                          n209 = Type Cast(x=w420) -> (*(type *) &x=w419:string)  [unwired: 1 in]
                          n210 = Concatenate Strings("Aw", w419) -> (w415:string)
                          n211 = local write "Command to Port"(w415) -> ()
                          n212 = call "write read Lens Driver.vi"("VISA resource name"=w423, "command"=w415, "Calibration"=w412, "error in (no error)"=w424) -> ("VISA resource name out"=w413:refnum<visa-resource-name>, "Calibration 2"=w417:T3, "OK"=w416:bool, "Data"=w414:string, "error out"=w425:errorcluster)  [unwired: 4 in, 3 out]
                          n213 = local write "VISA resource name out 2"(w413) -> ()
                          n214 = local write "Calibration 2"(w417) -> ()
                          n215 = local write "Data"(w414) -> ()
                          n216 = local write "OK"(w416) -> ()
                          "DPT INICIALES I" <- "Potencia inicial lente izquierdo"
                        }
                      }
                      n217 = local read "Parar adquisicion"() -> (w395:bool)
                    }
                  }
                  frame Error {
                  }
                }
                n218 = VISA Close(VISA resource name=w290, error in (no error)=w291) -> (error out=w293:errorcluster)
                n219 = call <vilib>:"Simple Error Handler.vi"("error in (no error)"=w293) -> ("error out"=→"error out 4":errorcluster)  [unwired: 4 in, 4 out]
              }
              frame 1 {
                # "Mensaje que pregunta si desea realizar el experimento\ncon un nuevo usuario o con el actual"
                # "Se vuelven 0 los valores del WL y de la potencia óptica y distancia"
                # "En esta opcion se activa el modo experimento"
                n220 = property on="Waveform length" class="WFChart (strict)"("History Data"=dbl[][] [[0.0]]) -> ()  [unwired: 2 in, 2 out]
                n221 = property on="Potencia optica y distancia" class="WFChart (strict)"("History Data"=dbl[][] [[0.0]]) -> ()  [unwired: 2 in, 2 out]
                n222 = Two Button Dialog(message="Con quien desea realizar los experimentos?", 1:"Nuevo voluntario" ("F button name (\"Cancel\")"), 2:"Voluntario actual" ("T button name (\"OK\")")) -> (T button?=w454:bool)
                n223 = flat-sequence {
                  tunnel: w454 -> [w467]
                  tunnel: [w466] -> w452
                  tunnel: w451 -> [w466]
                  tunnel: [w459] -> w439
                  tunnel: w438 -> [w459]
                  tunnel: [w477] -> w455
                  tunnel: [w479] -> w453
                  tunnel: w452 -> [w479]
                  tunnel: [w478] -> w449
                  tunnel: w448 -> [w478]
                  tunnel: [w476] -> w440
                  tunnel: w439 -> [w476]
                  tunnel: w455 -> [w491]
                  tunnel: w453 -> [w490]
                  tunnel: [w489] -> w450
                  tunnel: w449 -> [w488]
                  tunnel: [w487] -> w446
                  tunnel: [w486] -> w445
                  tunnel: [w485] -> w443
                  tunnel: [w484] -> w441
                  tunnel: w440 -> [w484]
                  tunnel: w446 -> [w537]
                  tunnel: w445 -> [w520]
                  tunnel: [w537] -> w444
                  tunnel: w443 -> [w523]
                  tunnel: [w516] -> w442
                  tunnel: w441 -> [w516]
                  tunnel: [w540] -> w447
                  tunnel: w444 -> [w540]
                  tunnel: w442 -> [w538]
                  frame #0 {
                    # "Se guardan los datos de un nuevo voluntario"
                    n224 = Not(x=w467) -> (.not. x?=w461:bool)
                    n225 = case shown="True" w461 {
                      tunnel: [w470 w475] -> w465
                      tunnel: [w469 w474] -> w464
                      tunnel: [w471 w473] -> w463
                      tunnel: [w468 w472] -> w462
                      frame False {
                        n226 = local read "Enfermedad visual"() -> (w470:string)
                        n227 = local read "Nombre"() -> (w471:string)
                        n228 = local read "Cedula"() -> (w468:string)
                        n229 = local read "Edad"() -> (w469:string)
                      }
                      frame True {
                        n230 = call "Registro voluntario"() -> ("Enfermedad visual"=w475:string, "Edad"=w474:string, "Cedula"=w472:string, "Nombre"=w473:string)  [unwired: 14 in, 2 out]
                      }
                    }
                    "Cedula" <- w462
                    "Nombre" <- w463
                    "Edad" <- w464
                    "Enfermedad visual" <- w465
                    n231 = local write "T button?"(FALSE ("T button?")) -> ()
                  }
                  frame #1 {
                    n232 = Two Button Dialog(message="Qué tipo de experimento desea realizar?", 1:"Nuevo Experimento" ("F button name (\"Cancel\")"), 2:"Experimento existente" ("T button name (\"OK\")")) -> (T button?=w480:bool)
                    n233 = Not(x=w480) -> (.not. x?=w477:bool)
                  }
                  frame #2 {
                    # "A partir de la seleccion del experimento, se obtiene la descripcion correspondiente que será guardada en el archivo"
                    n234 = case shown="False" w491 {
                      tunnel: w490 -> [w493 w511]
                      tunnel: [w493 w510] -> w489
                      tunnel: w488 -> [w495 w509]
                      tunnel: [w495 w508] -> w487
                      tunnel: [w496 w507] -> w486
                      tunnel: [w492 w506] -> w485
                      frame False {
                        n235 = call "Display Message to User"() -> ()  [unwired: 10 in, 2 out]
                        n236 = flat-sequence {
                          tunnel: [w497] -> w494
                          tunnel: w493 -> [w497]
                          tunnel: [w505] -> w496
                          tunnel: w495 -> [w504]
                          tunnel: ["Menu experimentos"] -> _
                          tunnel: w494 -> [w502]
                          tunnel: [w501] -> w492
                          frame #0 {
                            n237 = while {
                              stop <- w498 stop-if-true
                              # "El sistema se queda en el loop hasta que el usuario elija el experimento que desea realizar"
                              n238 = event shown="[0] \"Elegir menu Exp\": Value Change" {
                                selector: _ -> [_ _]
                                dyn-events: _ -> [_ _]
                                timeout: _ -> [_ _]
                                tunnel: [TRUE FALSE] -> w498
                                event "Elegir menu Exp": Value Change {
                                n239 = event-data() -> ()  [unwired: 1 in, 4 out]
                                }
                                event Timeout {
                                n240 = event-data() -> ()  [unwired: 1 in, 3 out]
                                }
                              }
                            }
                          }
                          frame #1 {
                            n241 = Index Array(array=w504, index="Menu experimentos") -> (element=w505:string)
                            n242 = Index Array(array=w502, index="Menu experimentos") -> (element=w501:string)
                          }
                        }
                        "Array" <- w493
                      }
                      frame True {
                        # "Se añade el nuevo experimento al menu de seleccion de experimentos"
                        # "Se guarda el nuevo experimento en el archivo que los contiene"
                        n243 = call "Nuevo experimento"() -> ("Descripcion"=w507:string, "Nombre"=w506:string)  [unwired: 16 in, 2 out]
                        n244 = Insert Into Array(array=w509, new element=w507) -> (w508:string[])  [unwired: 1 in]
                        n245 = Insert Into Array(array=w511, new element=w506) -> (w510:string[])  [unwired: 1 in]
                        n246 = property on="Menu experimentos" class="Ring (strict)"("Strings []"=w510) -> ()  [unwired: 2 in, 2 out]
                        n247 = Insert Into Array(array=string[] [], new element #1=w506, new element #2=w507) -> (w513:string[])  [unwired: 1 in]
                        n248 = call-poly <vilib>:"Write Delimited Spreadsheet.vi"("file path (dialog if empty)"=path "C:/Users/TGM1603/Documents/LabVIEW Data/Experimentos_realizados", "1D data"=w513, "append to file? (new file:F)"=TRUE) -> ()  [unwired: 11 in, 2 out]
                      }
                    }
                  }
                  frame #3 {
                    # "Se guardan los datos generales del experimento en el archivo de excel"
                    n249 = local read "factor decimacion"() -> (w519:i32)
                    n250 = local read "Enfermedad visual"() -> (w522:string)
                    n251 = local read "Cedula"() -> (w524:string)
                    n252 = local read "Edad"() -> (w521:string)
                    n253 = local read "Nombre"() -> (w525:string)
                    n254 = Get Date/Time In Seconds() -> (seconds since 1Jan1904=w536:timestamp)
                    n255 = Path To String(path="Carpeta") -> (string=w532:string)
                    n256 = Format Date/Time String(time format string (%c)="_%d-%m-%y_%H-%M", seconds (now)=w536) -> (date/time string=w534:string)  [unwired: 1 in]
                    n257 = Number To Fractional String(number=w519, precision (6)=i16 0) -> (F-format string=w518:string)  [unwired: 2 in]
                    n258 = local read "Cedula"() -> (w528:string)
                    n259 = Concatenate Strings(w532, "\\" ("string"), w528, w534, "_" ("string"), w523, ".xlsx" ("string")) -> (w530:string)
                    n260 = String To Path(string=w530) -> (path=w529:path)
                    "path" <- w529
                    n261 = call "MS Office Report"("Path to Save Report"=w529, "Cedula"=w524, "decimacion"=w518, "Edad"=w521, "Enfermedad"=w522, "Exp_nombre"=w523, "Experimento"=w520, "Nombre"=w525) -> ()  [unwired: 18 in, 2 out]
                    "Nombre 2" <- w523
                  }
                  frame #4 {
                    n262 = while {
                      shift-right: [w542] -> _
                      shift-left: enum16{"Inicio", "Tomar datos", ""}."Inicio" -> [w544]
                      tunnel: w538 -> [w541]
                      stop <- w543 stop-if-true
                      n263 = case shown="\"Tomar datos\"" w544 {
                        tunnel: [w545 w556] -> w542
                        tunnel: w541 -> [_ w551]
                        frame "Inicio", Default {
                          # "Se chequea si el usuario ha presionado el boton de comenzar el experimento. Si no lo ha hecho, se queda en este estado (0).\n Cuando lo presiona, pasa al estado de adquirir datios (1) ."
                          n264 = Select(t=enum16{"Inicio", "Tomar datos", ""}."Tomar datos", s="Iniciar experimento", f=enum16{"Inicio", "Tomar datos", ""}."Inicio") -> (s? t:f=w545:enum16{"Inicio", "Tomar datos", ""})
                        }
                        frame "Tomar datos" {
                          n265 = flat-sequence {
                            tunnel: [w649] -> w555
                            tunnel: [w648] -> w554
                            tunnel: [w647] -> w553
                            tunnel: [w646] -> w552
                            tunnel: w551 -> [w640]
                            tunnel: [w623] -> w550
                            tunnel: [w603] -> w549
                            tunnel: w555 -> [w954]
                            tunnel: w554 -> [w953]
                            tunnel: w553 -> [w952]
                            tunnel: w552 -> [w951]
                            tunnel: w550 -> [w948]
                            tunnel: w549 -> [w949]
                            tunnel: [enum16{"Inicio", "Tomar datos", ""}."Inicio"] -> w556
                            frame #0 {
                              w560 = 10123 items=["Finite Samples"=10178, "Continuous Samples"=10123, "Hardware Timed Single Point"=12522] ("sample mode")
                              w564 = 10083 items=["Default"=-1, "RSE"=10083, "NRSE"=10078, "Differential"=10106, "Pseudodifferential"=12529] ("input terminal configuration")
                              w589 = u16 0 items=["None", "Last Bit", "TermChar", "Break"] ("Serial Settings:End Mode for Writes")
                              w590 = u16 2 items=["None", "Last Bit", "TermChar"] ("Serial Settings:End Mode for Reads")
                              w614 = u16 0 items=["None", "Last Bit", "TermChar", "Break"] ("Serial Settings:End Mode for Writes")
                              w615 = u16 2 items=["None", "Last Bit", "TermChar"] ("Serial Settings:End Mode for Reads")
                              w638 = 100  # max queue size
                              # "[9] Se unen en una sola matriz los vectores de tiempo, distancia, potencia derecha y potencia izquierda."
                              # "[9]"
                              # "[12] Se unen en una sola matriz, los vectores de  tiempo de la señal EMG, amplitud de la señal EMG, tiempo de potencia óptica, distancia, potencia óptica derecha y potencia óptica izquierda, en ese orden."
                              # "[8]"
                              # "[7]"
                              # "[6]"
                              # "[5]"
                              # "Se usan registros de desplazamiento para concatenar en un solo vector los datos que se obtienen en cada iteracion. Así en \n[1] Se guarda la potencia del lente derecho.\n[2] Por medio de variables locales, se guarda la distancia que se obtuvo en el bloque de distancia.\n[3]  Por medio de variables locales, se guarda la potencia del lente izquierdo que se obtuvo en el bloque de control de potencia del lente izquierdo.\n[4] Se guarda el tiempo actual.\n[5] Se pasa el vector de de potencia derecha a variable a string con 2 cifras significativas. \n[6] Se ajusta el vector del tiempo para que se muestre un tiempo relativo, es decir, en donde el primer dato sea 0 y en los demas se aumente un dt.  Además, se pasa el vector a variable a string con 5 cifras significativas.\n[7] Se pasa el vector de de distancia a variable a string con 0 cifras significativas. \n[8] Se pasa el vector de de potencia izquierda a variable a string con 2 cifras significativas."
                              # "En esta cola se guarda los datos de la señal EMG\nEn el bloque de adquisición los añade al adquirirlos y  en el de procesamiento los elimina al procesarlos ."
                              # "Initialize VISA port with correct parameters"
                              # "Initialize VISA port with correct parameters"
                              # "Close VISA port after program stop. Otherwise this port is blocked."
                              # "Se adquiere la señal del circuito de adquisicion, en donde se define la frecuencia de muestreo y el factor de decimacion.\n[1] Se inicializa el canal de adquisicion\n[2] Se ajusta el canal para que lea muestras continuas y apartir de estas prooduzca waveform data.\n[3]  Se obtiene los datos de la señal: la amplitud Y, el tiempo de inicio y el delta t.\n[4] Se decima el vector de amplitud. \n[5] Se usan registros de desplazamiento para concatenenar en un solo vector los datos de la amplitud que se obtienen en cada iteración. \n[6] Se obtiene el vector del tiempo."
                              # "[11] Los vectores de amplitud y tiempo se transforman a formato texto con 4 y 5 cifras significativas respectivamente y se unen para formar un vector de 2 columnas."
                              # "[9] Se ajusta el vector del tiempo para que se muestre un tiempo relativo, es decir, en donde el primer dato sea 0 y en los demas se aumente un dt. \n[10] Se extrae el primer elemento del vector ya que este siempre es 0 y no aporta información"
                              # "[12]"
                              # "[11]"
                              # "[10]"
                              # "[9]"
                              # "[8] Se guarda la fecha/hora en que se inicio el experimento"
                              # "[7] Se usan registros de desplazamiento para concatenar en un solo vector los datos del tiempo que se obtienen en cada iteracion."
                              # "[1]"
                              n266 = while {
                                stop <- w676 stop-if-true
                                # "En este bloque se lleva a cabo la grabacion de video"
                                n267 = local read "Parar adquisicion"() -> (w671:bool)
                                n268 = call "grabarVideo.vi"("VideoMode"="Modo de video", "Quality"="Calidad", "Stop (F)"=w671, "Image Logging Path"="Carpeta archivo", "Frame Rate"="Frame Rate") -> ("Image Out"=→"Image Out":T1, "Stopped"=w676:bool)  [unwired: 20 in, 1 out]
                              }
                              n269 = local read "error in (no error)"() -> (w610:errorcluster)
                              n270 = local read "VISA resource name"() -> (w609:string)
                              n271 = local read "VISA resource name 2"() -> (w585:string)
                              n272 = call-poly "VISA Configure Serial Port"("VISA resource name"=w609, "timeout (10sec)"=u32 2000, "Enable Termination\nChar (T)"=FALSE ("Enable Termination\nChar (T)"), "baud rate (9600)"=u32 115200, "error in (no error)"=w610) -> ("VISA resource name out"=w619:refnum<visa-resource-name>, "error out"=w617:errorcluster)  [unwired: 9 in]
                              n273 = call-poly "VISA Configure Serial Port"("VISA resource name"=w585, "timeout (10sec)"=u32 2000, "Enable Termination\nChar (T)"=FALSE ("Enable Termination\nChar (T)"), "baud rate (9600)"=u32 115200, "error in (no error)"="error in (no error) 5") -> ("VISA resource name out"=w594:refnum<visa-resource-name>, "error out"=w592:errorcluster)  [unwired: 9 in]
                              n274 = property class="Instr"(reference=w619, error in=w617, "TermChar"=u8 10 ("Message Based Settings:Termination Character"), "ASRL End In"=w615, "ASRL End Out"=w614) -> (reference out=w618:refnum<visa-resource-name>, error out=w616:errorcluster)
                              n275 = property class="Instr"(reference=w594, error in=w592, "TermChar"=u8 10 ("Message Based Settings:Termination Character"), "ASRL End In"=w590, "ASRL End Out"=w589) -> (reference out=w593:refnum<visa-resource-name>, error out=w591:errorcluster)
                              n276 = VISA Set I/O Buffer Size(VISA resource name=w618, error in (no error)=w616) -> (VISA resource name out=w612:refnum<visa-resource-name>, error out=w611:errorcluster)  [unwired: 2 in]
                              n277 = VISA Set I/O Buffer Size(VISA resource name=w593, error in (no error)=w591) -> (VISA resource name out=w587:refnum<visa-resource-name>, error out=w586:errorcluster)  [unwired: 2 in]
                              n278 = VISA Flush I/O Buffer(VISA resource name=w612, error in (no error)=w611) -> (VISA resource name out=w608:refnum<visa-resource-name>, error out=w607:errorcluster)  [unwired: 1 in]
                              n279 = call-poly <vilib>:"DAQmx Create Virtual Channel.vi"("input terminal configuration"=w564, "physical channels"=tag "Dev1/ai0") -> ("task out"=w563:refnum<k21>, "error out"=w562:errorcluster)  [unwired: 12 in]
                              n280 = VISA Flush I/O Buffer(VISA resource name=w587, error in (no error)=w586) -> (VISA resource name out=w583:refnum<visa-resource-name>, error out=w582:errorcluster)  [unwired: 1 in]
                              n281 = invoke on="Parar adquisicion" class="Bool (strict)" method="Reinit To Default"() -> ()  [unwired: 3 in, 3 out]
                              n282 = Obtain Queue(max queue size (-1, unlimited)=w638, element data type="Cola tipo 2") -> (queue out=w637:refnum<queue>)  [unwired: 3 in, 2 out]
                              n283 = Enqueue Element(queue=w640, element=0.0) -> (queue out=w643:refnum<queue>)  [unwired: 2 in, 2 out]
                              n284 = call-poly <vilib>:"DAQmx Timing.vi"("task/channels in"=w563, "sample mode"=w560, "samples per channel"=1000, "rate"=1000.0, "error in"=w562) -> ("task out"=w558:refnum<k21>, "error out"=w557:errorcluster)  [unwired: 9 in]
                              n285 = call <vilib>:"DAQmx Start Task.vi"("task/channels in"=w558, "error in"=w557) -> ("task out"=w661:refnum<k21>, "error out"=w662:errorcluster)  [unwired: 12 in]
                              n286 = case shown="No Error" w582 {
                                tunnel: w582 -> [w692 w749]
                                tunnel: w583 -> [w691 w750]
                                tunnel: [w690 w749] -> w569
                                tunnel: [w689 w750] -> w568
                                tunnel: [w679 dbl[] [-30.0]] -> _
                                frame No Error {
                                w688 = 2 ("length (rest)")
                                # "Bloque de control del izquierdo. Se explica en el caso 0 de visualziación general"
                                # "Initialize Lens Driver"
                                n287 = local read "Calibration"() -> (w680:T3)
                                n288 = for {
                                tunnel: w691 -> [w746]
                                tunnel: [w743] -> w683
                                tunnel: string[] ["Start", "MwDA", "CrMA00", "CrMB00", "CrUA00", "CrUB00", "CrLA00", "CrLB00", "PwTA\u0002Ð\u0001@"] -> [w741] mode=indexing
                                tunnel: [w740] -> w682
                                shift-right: [w744] -> w684
                                shift-left: w680 -> [w745]
                                shift-right: [w742] -> w685
                                shift-left: w692 -> [w747]
                                n289 = call "write read Lens Driver.vi"("VISA resource name"=w746, "command"=w741, "Calibration"=w745, "error in (no error)"=w747) -> ("VISA resource name out"=w743:refnum<visa-resource-name>, "Calibration 2"=w744:T3, "Data"=w740:string, "error out"=w742:errorcluster)  [unwired: 4 in, 4 out]
                                }
                                n290 = String Subset(string=w682, offset (0)=w688, length (rest)=w688) -> (substring=w686:string)
                                n291 = Type Cast(type=u16 0 ("length (rest)"), x=w686) -> (*(type *) &x=w681:u16)
                                n292 = local write "ID"(w681) -> ()
                                n293 = while {
                                tunnel: [w697] -> w690
                                tunnel: [w698] -> w689
                                tunnel: w685 -> [w703]
                                tunnel: w684 -> [w702]
                                tunnel: w683 -> [w701]
                                shift-right: [w694] -> w679
                                shift-left: _ -> [w695]
                                stop <- w696 stop-if-true
                                # "When Send command is true, Current Ch A is sent to the Lens Driver, in the correct format. If answer exists it is displayed in Data. The update rate of the while loop is 2ms."
                                n294 = case shown="True" TRUE ("Send command") {
                                tunnel: [w709 w732] -> w697
                                tunnel: w703 -> [w709 w731]
                                tunnel: w702 -> [_ w712]
                                tunnel: w701 -> [w708 w730]
                                tunnel: [w708 w723] -> w698
                                tunnel: [dbl[] [-20.0] w722] -> w694
                                tunnel: w695 -> [_ w721]
                                frame False {
                                }
                                frame True {
                                n295 = local read "Potencia inicial lente izquierdo"() -> (w720:dbl)
                                n296 = local read "DPT dif."() -> (w719:dbl)
                                n297 = Add(x=w719, y=w720) -> (x+y=w715:dbl)
                                n298 = Absolute Value(x=w715) -> (abs(x)=w717:dbl)
                                n299 = Greater Or Equal?(x=6.0, y=w717) -> (x >= y?=w716:bool)
                                n300 = case shown="False" w716 {
                                tunnel: w715 -> [w735 w739]
                                tunnel: [w733 w739] -> w713
                                frame False {
                                n301 = Greater Or Equal?(x=u16 0, y=w735) -> (x >= y?=w736:bool)
                                n302 = case shown="False" w736 {
                                tunnel: [i16 6 ("x") i16 -6 ("x")] -> w733
                                frame False {
                                }
                                frame True {
                                }
                                }
                                }
                                frame True {
                                }
                                }
                                "Potencia izquierdo" <- w713
                                n303 = Unbundle By Name(w712) -> ("Max Current A"=w711:dbl)
                                n304 = call "potencia a corriente.vi"("Max current A"=w711, "Potencia"=w713) -> ("Corriente"=w714:dbl)
                                n305 = To Word Integer(number=w714) -> (16bit integer=w729:i16)
                                n306 = Type Cast(x=w729) -> (*(type *) &x=w728:string)  [unwired: 1 in]
                                n307 = Concatenate Strings("Aw", w728) -> (w725:string)
                                n308 = local write "Command to Port"(w725) -> ()
                                n309 = call "write read Lens Driver.vi"("VISA resource name"=w730, "command"=w725, "Calibration"=w712, "error in (no error)"=w731) -> ("VISA resource name out"=w723:refnum<visa-resource-name>, "Calibration 2"=w727:T3, "OK"=w726:bool, "Data"=w724:string, "error out"=w732:errorcluster)  [unwired: 4 in, 3 out]
                                n310 = local write "VISA resource name 2"(w723) -> ()
                                n311 = local write "Calibration 2"(w727) -> ()
                                n312 = local write "Data"(w724) -> ()
                                n313 = local write "OK"(w726) -> ()
                                n314 = Build Array (concatenate)(w721, w713) -> (w722:dbl[])
                                }
                                }
                                n315 = Wait Until Next ms Multiple(millisecond multiple=u32 10) -> ()  [unwired: 1 out]
                                n316 = local read "Parar adquisicion"() -> (w696:bool)
                                n317 = event shown="[0] \"Restablecer Iniciales\": Value Change" {
                                selector: _ -> [_ _]
                                dyn-events: _ -> [_ _]
                                timeout: 100 -> [_ _]
                                event "Restablecer Iniciales": Value Change {
                                n318 = event-data() -> ()  [unwired: 1 in, 3 out]
                                n319 = local read "Potencia inicial lente izquierdo"() -> (w704:dbl)
                                n320 = local read "Potencia inicial lente derecho"() -> (w705:dbl)
                                n321 = local write "Potencia izquierdo"(w704) -> ()
                                n322 = local write "Potencia derecho"(w705) -> ()
                                n323 = local write "DPT dif."(0.0 ("DPT dif.")) -> ()
                                }
                                event Timeout {
                                n324 = event-data() -> ()  [unwired: 1 in, 3 out]
                                }
                                }
                                }
                                }
                                frame Error {
                                }
                              }
                              n325 = case shown="No Error" w607 {
                                tunnel: w607 -> [w772 w868]
                                tunnel: w608 -> [w771 w869]
                                tunnel: [w770 w868] -> w635
                                tunnel: [w769 w869] -> w634
                                tunnel: [w758 dbl[] [-1.0]] -> w627
                                tunnel: [w757 dbl[] [-30.0]] -> w575
                                tunnel: [w756 u32[] [0]] -> w605
                                tunnel: [w754 dbl[] [-30.0]] -> w578
                                frame No Error {
                                w768 = 2 ("length (rest)")
                                # "Bloque de control del lente derecho. Se explica en el caso 0 de visualziación general"
                                # "Initialize Lens Driver"
                                n326 = local read "Calibration"() -> (w760:T3)
                                n327 = for {
                                tunnel: w771 -> [w862]
                                tunnel: [w859] -> w763
                                tunnel: string[] ["Start", "MwDA", "CrMA00", "CrMB00", "CrUA00", "CrUB00", "CrLA00", "CrLB00", "PwTA\u0002Ð\u0001@"] -> [w857] mode=indexing
                                tunnel: [w856] -> w762
                                shift-right: [w860] -> w764
                                shift-left: w760 -> [w861]
                                shift-right: [w858] -> w765
                                shift-left: w772 -> [w863]
                                n328 = call "write read Lens Driver.vi"("VISA resource name"=w862, "command"=w857, "Calibration"=w861, "error in (no error)"=w863) -> ("VISA resource name out"=w859:refnum<visa-resource-name>, "Calibration 2"=w860:T3, "Data"=w856:string, "error out"=w858:errorcluster)  [unwired: 4 in, 4 out]
                                }
                                n329 = String Subset(string=w762, offset (0)=w768, length (rest)=w768) -> (substring=w766:string)
                                n330 = Type Cast(type=u16 0 ("length (rest)"), x=w766) -> (*(type *) &x=w761:u16)
                                n331 = local write "ID"(w761) -> ()
                                n332 = while {
                                tunnel: [w790] -> w770
                                tunnel: [w791] -> w769
                                tunnel: w765 -> [w796]
                                tunnel: w764 -> [w795]
                                tunnel: w763 -> [w794]
                                shift-right: [w777] -> w758
                                shift-left: dbl[] [0.0] -> [w778]
                                shift-right: [w785] -> w757
                                shift-left: dbl[] [0.0] -> [w788]
                                shift-right: [w784] -> w756
                                shift-left: u32[] [0] -> [w787]
                                shift-right: [w775] -> w754
                                shift-left: dbl[] [0.0] -> [w774]
                                stop <- w789 stop-if-true
                                # "[4]"
                                # "[3]"
                                # "[2]"
                                # "When Send command is true, Current Ch A is sent to the Lens Driver, in the correct format. If answer exists it is displayed in Data. The update rate of the while loop is 2ms."
                                n333 = Wait Until Next ms Multiple(millisecond multiple=u32 10) -> ()  [unwired: 1 out]
                                n334 = case shown="True" TRUE ("Send command") {
                                tunnel: [w803 w822] -> w790
                                tunnel: w796 -> [w803 w821]
                                tunnel: w795 -> [_ w806]
                                tunnel: w794 -> [w802 w820]
                                tunnel: [w802 w812] -> w791
                                tunnel: [dbl[] [-20.0] w811] -> w785
                                tunnel: w788 -> [_ w810]
                                frame False {
                                }
                                frame True {
                                # "[1]"
                                n335 = local read "number"() -> (w817:u32)
                                n336 = local read "Potencia inicial lente derecho"() -> (w809:dbl)
                                n337 = case shown="2" w817 {
                                tunnel: [w823 w832 w847] -> w808
                                tunnel: w809 -> [w825 w827 w842]
                                tunnel: w809 -> [_ w826 w841]
                                frame 0, Default {
                                n338 = local read "DPT dif."() -> (w824:dbl)
                                n339 = Add(x=w825, y=w824) -> (x+y=w823:dbl)
                                }
                                frame 1 {
                                n340 = local read "DPT dif."() -> (w828:dbl)
                                n341 = Add(x=w827, y=w828) -> (x+y=w829:dbl)
                                n342 = Less Or Equal?(x=w829, y=6.0) -> (x <= y?=w831:bool)
                                n343 = case shown="True" w831 {
                                tunnel: [w834 w838] -> w832
                                tunnel: w826 -> [w833 w837]
                                frame False {
                                n344 = local read "DPT dif."() -> (w835:dbl)
                                n345 = Add(x=w833, y=w835) -> (x+y=w834:dbl)
                                }
                                frame True {
                                n346 = local read "DPT dif."() -> (w839:dbl)
                                n347 = local read "Incremento"() -> (w836:dbl)
                                n348 = Add(x=w839, y=w836) -> (x+y=w840:dbl)
                                n349 = local write "DPT dif."(w840) -> ()
                                n350 = Add(x=w837, y=w840) -> (x+y=w838:dbl)
                                }
                                }
                                }
                                frame 2 {
                                n351 = local read "DPT dif."() -> (w846:dbl)
                                n352 = Add(x=w846, y=w842) -> (x+y=w843:dbl)
                                n353 = Greater Or Equal?(x=w843, y=-6.0) -> (x >= y?=w844:bool)
                                n354 = case shown="True" w844 {
                                tunnel: [w849 w853] -> w847
                                tunnel: w841 -> [w848 w852]
                                frame False {
                                n355 = local read "DPT dif."() -> (w850:dbl)
                                n356 = Add(x=w848, y=w850) -> (x+y=w849:dbl)
                                }
                                frame True {
                                n357 = local read "DPT dif."() -> (w855:dbl)
                                n358 = local read "Incremento"() -> (w851:dbl)
                                n359 = Subtract(x=w855, y=w851) -> (x-y=w854:dbl)
                                n360 = local write "DPT dif."(w854) -> ()
                                n361 = Add(x=w852, y=w854) -> (x+y=w853:dbl)
                                }
                                }
                                }
                                }
                                "Potencia derecho" <- w808
                                n362 = Unbundle By Name(w806) -> ("Max Current A"=w805:dbl)
                                n363 = call "potencia a corriente.vi"("Max current A"=w805, "Potencia"=w808) -> ("Corriente"=w807:dbl)
                                n364 = To Word Integer(number=w807) -> (16bit integer=w819:i16)
                                n365 = Type Cast(x=w819) -> (*(type *) &x=w818:string)  [unwired: 1 in]
                                n366 = Concatenate Strings("Aw", w818) -> (w814:string)
                                n367 = local write "Command to Port"(w814) -> ()
                                n368 = call "write read Lens Driver.vi"("VISA resource name"=w820, "command"=w814, "Calibration"=w806, "error in (no error)"=w821) -> ("VISA resource name out"=w812:refnum<visa-resource-name>, "Calibration 2"=w816:T3, "OK"=w815:bool, "Data"=w813:string, "error out"=w822:errorcluster)  [unwired: 4 in, 3 out]
                                n369 = local write "VISA resource name out"(w812) -> ()
                                n370 = local write "Calibration 2"(w816) -> ()
                                n371 = local write "Data"(w813) -> ()
                                n372 = local write "OK"(w815) -> ()
                                n373 = Build Array (concatenate)(w810, w808) -> (w811:dbl[])
                                }
                                }
                                n374 = local read "Parar adquisicion"() -> (w789:bool)
                                n375 = local read "Potencia izquierdo"() -> (w773:dbl)
                                n376 = local read "Distancia"() -> (w786:u32)
                                n377 = property on="Potencia optica y distancia" class="WFChart (strict)"("YScale.ScaleFit"="Auto scale Y") -> ()  [unwired: 2 in, 2 out]
                                n378 = Get Date/Time In Seconds() -> (seconds since 1Jan1904=w779:timestamp)
                                n379 = To Double Precision Float(number=w779) -> (double precision float=w776:dbl)
                                n380 = property on="Potencia optica y distancia" class="WFChart (strict)"("XScale.ScaleFit"="Auto scale X") -> ()  [unwired: 2 in, 2 out]
                                n381 = Build Array (concatenate)(w778, w776) -> (w777:dbl[])
                                n382 = case shown="0, Default" "Auto scale Y" {
                                frame 0, Default {
                                n383 = property on="Potencia optica y distancia" class="WFChart (strict)"("YScale.Maximum"="Escala Y max") -> ()  [unwired: 2 in, 2 out]
                                n384 = property on="Potencia optica y distancia" class="WFChart (strict)"("YScale.Minimum"="Escala Y min") -> ()  [unwired: 2 in, 2 out]
                                }
                                frame 1 {
                                }
                                }
                                n385 = Build Array (concatenate)(w774, w773) -> (w775:dbl[])
                                n386 = Build Array (concatenate)(w787, w786) -> (w784:u32[])
                                n387 = case shown="0, Default" "Auto scale X" {
                                frame 0, Default {
                                n388 = property on="Potencia optica y distancia" class="WFChart (strict)"("XScale.Maximum"="Escala X max") -> ()  [unwired: 2 in, 2 out]
                                n389 = property on="Potencia optica y distancia" class="WFChart (strict)"("XScale.Minimum"="Escala X min") -> ()  [unwired: 2 in, 2 out]
                                }
                                frame 1 {
                                }
                                }
                                n390 = Build Array(w785, w784) -> (w783:dbl[][])
                                n391 = Transpose 2D Array(2D array=w783) -> (transposed array=→"Potencia optica y distancia":dbl[][])
                                }
                                }
                                frame Error {
                                }
                              }
                              n392 = while {
                                tunnel: w643 -> [w901]
                                shift-right: [w903] -> _
                                shift-left: dbl[] [0.0] -> [w909]
                                shift-right: [w902] -> _
                                shift-left: u32[] [0] -> [w904]
                                tunnel: [w901] -> w641
                                tunnel: w637 -> [w893]
                                stop <- w892 stop-if-true
                                # "Bloque de procesamiento.  Se explica en el caso 0 de visualización general"
                                n393 = local read "WL"() -> (w900:dbl)
                                n394 = local read "Parar adquisicion"() -> (w892:bool)
                                n395 = local read "Limite superior WL"() -> (w897:dbl)
                                n396 = call "waveform_length.vi"("WL"=w900, "Cola WL"=w901, "Datos entrada"=w893) -> ("WL 2"=w908:dbl)
                                n397 = local read "Limite inferior WL"() -> (w899:dbl)
                                n398 = local write "WL"(w908) -> ()
                                n399 = Build Array (concatenate)(w909, w908) -> (w903:dbl[])
                                n400 = In Range and Coerce(upper limit=w897, x=w908, lower limit=w899) -> (In Range?=w906:bool)  [unwired: 1 out]
                                n401 = Greater?(x=w908, y=w897) -> (0:w907:bool)
                                n402 = local read "Escala autom. X"() -> (w894:u8)
                                n403 = local read "Escala autom. Y"() -> (w895:u8)
                                n404 = Build Array(w907, w906) -> (w905:bool[])
                                n405 = Boolean Array To Number(Boolean array=w905) -> (number=w898:u32)
                                n406 = local write "number"(w898) -> ()
                                n407 = Build Array (concatenate)(w904, w898) -> (w902:u32[])
                                n408 = Build Array(w903, w902) -> (w896:dbl[][])
                                n409 = Transpose 2D Array(2D array=w896) -> (transposed array=w891:dbl[][])
                                n410 = local write "Waveform length"(w891) -> ()
                                n411 = property on="Waveform length" class="WFChart (strict)"("XScale.ScaleFit"=w894) -> ()  [unwired: 2 in, 2 out]
                                n412 = property on="Waveform length" class="WFChart (strict)"("YScale.ScaleFit"=w895) -> ()  [unwired: 2 in, 2 out]
                                n413 = case shown="0, Default" w895 {
                                frame 0, Default {
                                n414 = local read "Maximo escala Y"() -> (w913:dbl)
                                n415 = local read "Minimo escala Y"() -> (w912:dbl)
                                n416 = property on="Waveform length" class="WFChart (strict)"("YScale.Maximum"=w913) -> ()  [unwired: 2 in, 2 out]
                                n417 = property on="Waveform length" class="WFChart (strict)"("YScale.Minimum"=w912) -> ()  [unwired: 2 in, 2 out]
                                }
                                frame 1 {
                                }
                                }
                                n418 = case shown="0, Default" w894 {
                                frame 0, Default {
                                n419 = local read "Minimo escala X"() -> (w911:dbl)
                                n420 = local read "Maximo escala X"() -> (w910:dbl)
                                n421 = property on="Waveform length" class="WFChart (strict)"("XScale.Minimum"=w911) -> ()  [unwired: 2 in, 2 out]
                                n422 = property on="Waveform length" class="WFChart (strict)"("XScale.Maximum"=w910) -> ()  [unwired: 2 in, 2 out]
                                }
                                frame 1 {
                                }
                                }
                              }
                              n423 = while {
                                tunnel: w661 -> [w943]
                                tunnel: [w941] -> w651
                                shift-right: [w939] -> w650
                                shift-left: w662 -> [w942]
                                tunnel: [w934] -> w670
                                shift-right: [w933] -> w648
                                shift-left: _ -> [w932]
                                shift-right: [w923] -> w653
                                shift-left: dbl[] [0.0] -> [w928]
                                shift-right: [w924] -> w658
                                shift-left: dbl[] [0.0] -> [w925]
                                tunnel: w637 -> [w916]
                                i -> [w935]
                                stop <- w938 stop-if-true
                                w937 = 10.0  # timeout (s)
                                # "[7]"
                                # "[6]"
                                # "[5]"
                                # "[4]"
                                # "[3]"
                                # "[2]"
                                n424 = local read "Parar adquisicion"() -> (w919:bool)
                                n425 = call-poly <vilib>:"DAQmx Read.vi"("task/channels in"=w943, "timeout"=w937, "error in"=w942) -> ("task out"=w941:refnum<k21>, "data"=w929:waveform(dbl)[], "error out"=w939:errorcluster)  [unwired: 10 in]
                                n426 = Unbundle By Name(w939) -> ("status"=w940:bool)
                                n427 = Or(x=w940, y=w919) -> (x .or. y?=w938:bool)
                                n428 = local write "Senal EMG"(w929) -> ()
                                n429 = call-poly <vilib>:"Index Waveform Array.vi"("index"=0, "waveform array"=w929) -> ("waveform"=w927:waveform(dbl))  [unwired: 8 in, 1 out]
                                n430 = Unbundle By Name(w927) -> ("Y"=w917:dbl[], "t0"=w934:timestamp)  [unwired: 1 out]
                                n431 = call-poly <vilib>:"Decimate (continuous).vi"("averaging"=TRUE, "decimating factor"="factor decimacion", "X"=w917) -> ("Decimated Array"=w914:dbl[])  [unwired: 7 in, 1 out]
                                n432 = Lossy Enqueue Element(queue=w916, element=w914) -> ()  [unwired: 1 in, 4 out]
                                n433 = Build Array (concatenate)(w928, w914) -> (w923:dbl[])
                                n434 = case shown="1" w935 {
                                tunnel: w934 -> [_ w947]
                                tunnel: [w945 w946] -> w933
                                tunnel: w932 -> [w945 _]
                                frame 0, Default {
                                }
                                frame 1 {
                                # "[8]"
                                n435 = Format Date/Time String(seconds (now)=w947) -> (date/time string=w946:string)  [unwired: 2 in]
                                }
                                }
                                n436 = local read "factor decimacion"() -> (w920:i32)
                                n437 = call-poly <vilib>:"Get Waveform Time Array.vi"("waveform in"=w927) -> ("X array"=w926:timestamp[])  [unwired: 9 in, 1 out]
                                n438 = event shown="[0] \"Ganancia\": Value Change" {
                                selector: _ -> [_ _]
                                dyn-events: _ -> [_ _]
                                timeout: 1 -> [_ _]
                                tunnel: "Ganancia" -> [w944 _]
                                event "Ganancia": Value Change {
                                n439 = event-data() -> ()  [unwired: 1 in, 4 out]
                                n440 = call "Ganancia programable.vi"("MOSI data"=w944) -> ()
                                }
                                event Timeout {
                                n441 = event-data() -> ()  [unwired: 1 in, 3 out]
                                }
                                }
                                n442 = To Double Precision Float(number=w926) -> (double precision float=w922:dbl[])
                                n443 = call-poly <vilib>:"Decimate (single shot).vi"("decimating factor"=w920, "X"=w922) -> ("Decimated Array"=w921:dbl[])  [unwired: 8 in, 1 out]
                                n444 = Build Array (concatenate)(w925, w921) -> (w924:dbl[])
                              }
                              n445 = call <vilib>:"DAQmx Clear Task.vi"("task in"=w651, "error in"=w650) -> ()  [unwired: 13 in, 1 out]
                              n446 = Index Array(array=w658, index=1) -> (element=w657:dbl)
                              n447 = Flush Queue(queue=w641) -> ()  [unwired: 1 in, 3 out]
                              n448 = Subtract(x=w658, y=w657) -> (x-y=w655:dbl[])
                              n449 = Delete From Array(array=w653, index=0) -> (array with subset deleted=w665:dbl[])  [unwired: 1 in, 1 out]
                              n450 = while {
                                shift-right: [w870] -> _
                                shift-left: _ -> [w871]
                                stop <- w875 stop-if-true
                                # "Este bloque adquiere la distancia (se explica en el caso 0 (visualizacion general)"
                                n451 = call "meididor de distancia archivo adicional.vi"() -> ("error out"=w878:errorcluster, "task out"=w879:refnum<k21>)  [unwired: 10 in]
                                n452 = call "DAQ Assistant2"("timeout (s)"=0.05) -> ("data"=w888:dynamicdata, "error out"=w876:errorcluster)  [unwired: 16 in, 1 out]
                                n453 = call <vilib>:"DAQmx Start Task.vi"("task/channels in"=w879, "error in"=w878) -> ("task out"=w882:refnum<k21>, "error out"=w883:errorcluster)  [unwired: 12 in]
                                n454 = call <vilib>:"DAQmx Is Task Done.vi"("task/channels in"=w882, "error in"=w883) -> ("task out"=w880:refnum<k21>, "error out"=w881:errorcluster)  [unwired: 11 in, 1 out]
                                n455 = Wait (ms)(milliseconds to wait=u32 200) -> ()  [unwired: 1 out]
                                n456 = call <vilib>:"Clear Errors.vi"("error in (no error)"=w876) -> ()  [unwired: 5 in, 2 out]
                                n457 = local read "Parar adquisicion"() -> (w875:bool)
                                n458 = call <vilib>:"DAQmx Clear Task.vi"("task in"=w880, "error in"=w881) -> ()  [unwired: 13 in, 1 out]
                                n459 = Multiply(x=1000000.0, y=w888) -> (x*y=w886:dynamicdata)
                                n460 = Divide(x=w886, y=58.0) -> (x/y=w872:dynamicdata)
                                n461 = Equal?(x=w872, y=0.0) -> (x = y?=w874:dynamicdata)
                                n462 = case shown="True" w874 {
                                tunnel: [w889 w890] -> w870
                                tunnel: w872 -> [w889 _]
                                tunnel: w871 -> [_ w890]
                                frame False {
                                }
                                frame True {
                                }
                                }
                                n463 = local write "Distancia"(w870) -> ()
                              }
                              n464 = Delete From Array(array=w655, index=0) -> (array with subset deleted=w664:dbl[])  [unwired: 1 in, 1 out]
                              n465 = local read "path"() -> (w649:path)
                              n466 = Format Date/Time String(seconds (now)=w670) -> (date/time string=w647:string)  [unwired: 2 in]
                              n467 = Number To Fractional String(use system decimal point (T)=FALSE, number=w665, precision (6)=i16 4) -> (F-format string=w601:string[])  [unwired: 1 in]
                              n468 = Number To Fractional String(use system decimal point (T)=FALSE, number=w664, precision (6)=i16 5) -> (F-format string=w602:string[])  [unwired: 1 in]
                              n469 = Build Array(w602, w601) -> (w663:string[][])
                              n470 = Transpose 2D Array(2D array=w663) -> (transposed array=w646:string[][])
                              n471 = Delete From Array(array=w575, index=0) -> (array with subset deleted=w574:dbl[])  [unwired: 1 in, 1 out]
                              n472 = Delete From Array(array=w605, index=0) -> (array with subset deleted=w571:u32[])  [unwired: 1 in, 1 out]
                              n473 = Index Array(array=w627, index=1) -> (element=w632:dbl)
                              n474 = Delete From Array(array=w578, index=0) -> (array with subset deleted=w577:dbl[])  [unwired: 1 in, 1 out]
                              n475 = VISA Close(VISA resource name=w568, error in (no error)=w569) -> (error out=w567:errorcluster)
                              n476 = Subtract(x=w627, y=w632) -> (x-y=w626:dbl[])
                              n477 = Number To Fractional String(use system decimal point (T)=FALSE, number=w574, precision (6)=i16 2) -> (F-format string=w598:string[])  [unwired: 1 in]
                              n478 = VISA Close(VISA resource name=w634, error in (no error)=w635) -> (error out=w636:errorcluster)
                              n479 = call <vilib>:"Simple Error Handler.vi"("error in (no error)"=w567) -> ("error out"=w566:errorcluster)  [unwired: 4 in, 4 out]
                              n480 = Number To Fractional String(number=w571, precision (6)=i16 0) -> (F-format string=w599:string[])  [unwired: 2 in]
                              n481 = Delete From Array(array=w626, index=0) -> (array with subset deleted=w631:dbl[])  [unwired: 1 in, 1 out]
                              n482 = call <vilib>:"Simple Error Handler.vi"("error in (no error)"=w636) -> ("error out"=w633:errorcluster)  [unwired: 4 in, 4 out]
                              n483 = Number To Fractional String(use system decimal point (T)=FALSE, number=w577, precision (6)=i16 2) -> (F-format string=w579:string[])  [unwired: 1 in]
                              n484 = local write "error out"(w633) -> ()
                              n485 = local write "error out"(w566) -> ()
                              n486 = Number To Fractional String(use system decimal point (T)=FALSE, number=w631, precision (6)=i16 5) -> (F-format string=w600:string[])  [unwired: 1 in]
                              n487 = Build Array(w602, w601, w600, w599, w598, w579) -> (w572:string[][])
                              n488 = Transpose 2D Array(2D array=w572) -> (transposed array=w603:string[][])
                              n489 = Build Array(w600, w599, w598, w579) -> (w623:string[][])
                            }
                            frame #1 {
                              # "[13]"
                              # "[13] En esta case structure, se decide que datos se van a guardar. Esto lo hace el SUBVI llamado guardar datos de amplitud y tiempo."
                              n490 = Transpose 2D Array(2D array=w948) -> (transposed array=w950:string[][])
                              n491 = call <vilib>:"Three Button Dialog.vi"("Right Button Text (\"Cancel\")"="Señal EMG, potencia optica y distancia" ("Right Button Text (\"Cancel\")"), "Center Button Text (\"No\")"="Potencia optica y distancia" ("Center Button Text (\"No\")"), "Left Button Text (\"Yes\")"="Señal EMG" ("Left Button Text (\"Yes\")"), "message"="Elija que datos desea guardar") -> ("Which Button?"=w955:T4)  [unwired: 7 in]
                              n492 = case shown="\"Center Button\"" w955 {
                                tunnel: w954 -> [w964 w969 w972]
                                tunnel: w953 -> [w963 w968 w973]
                                tunnel: w952 -> [w962 w967 w974]
                                tunnel: w951 -> [w961 _ _]
                                tunnel: w950 -> [_ w966 _]
                                tunnel: w949 -> [_ _ w970]
                                frame "Left Button", Default {
                                # "Se guarda solo la señal EMG y su tiempo de adquisición."
                                n493 = call "Guardar datos de Amplitud y Tiempo.vi"("path"=w964, "Hora inicio"=w963, "Hora fin"=w962, "Datos experimento"=w961, "column headers"=string[] ["Tiempo(s)", "Amplitud(V)"]) -> ()  [unwired: 1 in]
                                }
                                frame "Center Button" {
                                # "Se guarda la potenica del lente derecho, del lente izquierdo, la distancia y el tiempo de estas variables."
                                n494 = call "Guardar datos de Amplitud y Tiempo.vi"("path"=w969, "Hora inicio"=w968, "Hora fin"=w967, "Datos experimento"=w966, "column headers"=string[] ["Tiempo(s)", "Distancia (cm)", "Potencia Optica derecho", "Potencia optica izquierdo"]) -> ()  [unwired: 1 in]
                                }
                                frame "Right Button" {
                                # "Se guarda el tiempo de adquisición así como la amplitud de la señal EMG,  la potenica del lente derecho, del lente izquierdo, la distancia y el tiempo de estas variables."
                                n495 = call "Guardar datos de Amplitud y Tiempo.vi"("path"=w972, "Hora inicio"=w973, "Hora fin"=w974, "Datos experimento"=w970, "column headers"=string[] ["Tiempo EMG(s)", "Amplitud(V)", "Tiempo DPT(s)", "Distancia (cm)", "Potencia optica derecho", "Potencia optica izquierdo"]) -> ()  [unwired: 1 in]
                                }
                              }
                            }
                            frame #2 {
                              # "Si el usuario desea repetir el experimento se vuelve al estado inicio en donde se espera que comience el experimento. De lo contrario se sale del loop y vuelve al menu principal."
                              n496 = Two Button Dialog(message="¿Desea repetir el experimento?", 1:"No" ("F button name (\"Cancel\")"), 2:"Si" ("T button name (\"OK\")")) -> (T button?=w977:bool)
                              n497 = Not(x=w977) -> (.not. x?=→"T button?":bool)
                            }
                          }
                        }
                      }
                      n498 = local read "T button?"() -> (w543:bool)
                    }
                  }
                }
                "Array 2" <- w451
              }
            }
          }
          event Timeout {
            n499 = event-data() -> ()  [unwired: 1 in, 3 out]
          }
        }
        "Array 3" <- w31
      }
      "Array 4" <- w22
    }
  }
